vi "Auto_calibrate.vi"(3 "Mode":T4, 5 "Traverse line":T5 {"Carrier_2 Q (l/min)" format="%#.2f"; "Row Duration (mins)" format="%#.1f"; "Row No" min=0; "Trace Gas Concentration (%)" min=0.0 format="%#_4f"; "Carrier_1 Q (l/min)" format="%#.2f"; "Tunnel Speed" format="%#.2f"; "Start X" format="%#.2f"; "Start Y" format="%#.2f"; "Start Z" format="%#.2f"; "End X" format="%#.2f"; "End Y" format="%#.2f"; "End Z" format="%#.2f"; "Averaging time (min)" min=0.0 format="%#.2f"}) -> (0 "Error Messages":string, 1 "Status":T2, 2 "Traverse Out":T5 {"Carrier_2 Q (l/min)" format="%#.2f"; "Row Duration (mins)" format="%#.1f"; "Row No" min=0; "Trace Gas Concentration (%)" min=0.0 format="%#_4f"; "Carrier_1 Q (l/min)" format="%#.2f"; "Tunnel Speed" format="%#.2f"; "Start X" format="%#.2f"; "Start Y" format="%#.2f"; "Start Z" format="%#.2f"; "End X" format="%#.2f"; "End Y" format="%#.2f"; "End Z" format="%#.2f"; "Averaging time (min)" min=0.0 format="%#.2f"})   [LabVIEW 2014]
uses:
  Gen Trav/Traverse_cluster.ctl
  Gen Trav/Spacing.ctl
  Controls/Multi_run_mode.ctl
  Controls/User_Specific_mode.ctl
  Controls/Auto_Calib_Type.ctl
  Gen Trav/Multi_Run_Status.ctl
  Controls/Auto_Calib_Case.ctl
  File/Setup_Filetype.ctl
  Calibration/Calib_mode.ctl
  ADAM Client/Sub VIs/ADAM Controls/Valco_valve_ph.ctl
  ADAM Client/Sub VIs/ADAM Controls/Client_Source_Status.ctl
  Controls/Setup.ctl
  Controls/Post_Process.ctl
  Controls/Save_Data.ctl
  Controls/App_Global.ctl
  <vilib>/Analysis/baseanly.llb/Mean (DBL).vi
  Globals/Preference_global.vi
  Globals/Meas_global.vi
  Globals/Calib_global.vi
  Globals/Trav_pos_global.vi
  Globals/Gas_management_global.vi
  Globals/Extra_Commands_Global.vi
  <vilib>/Analysis/NI_AALBase.lvlib
  <vilib>/Analysis/NI_AALPro.lvlib
panel:
  out "Mix_own_Calib_Gases":bool
  out "Slope":dbl[](array[numeric])
  out "Minimum St Dev":dbl[](array[numeric])
  out "Wait factor":dbl
  out "Orig Calib file string":string
  out "Concentrations":dbl[](array[numeric])
  out "FFID St Dev":dbl[][](array[numeric]) format="%.2f"
  in  "Clear Calib History":bool
  out "Coefficients":dbl[][](array[numeric]) format="%.2f"
  out "Currently in Case":T1
  out "Valve position":dbl format="%.2f"
  out "Currently On":i32
  out "Values":dbl[][](array[numeric]) format="%.2f"
  out "FF Indexes":i16[](array[numeric])
  out "Ch No's":i16[](array[numeric])
  out "No of Calib Points":i32
  out "Root Name":string[](array[string])
  out "Calibration varying":T3
  in  "stop":bool
  out "New Calib Filenames":path[](array[path])
  # "Specific Argument Options\n      Tunnel Speed;1;2;3;4\nOR  Traverse Position\nOR   Concentration"
  # "X           Y            Z"
  # "Start"
  # "End"
  # "X           Y            Z"
  # "Start"
  # "End"
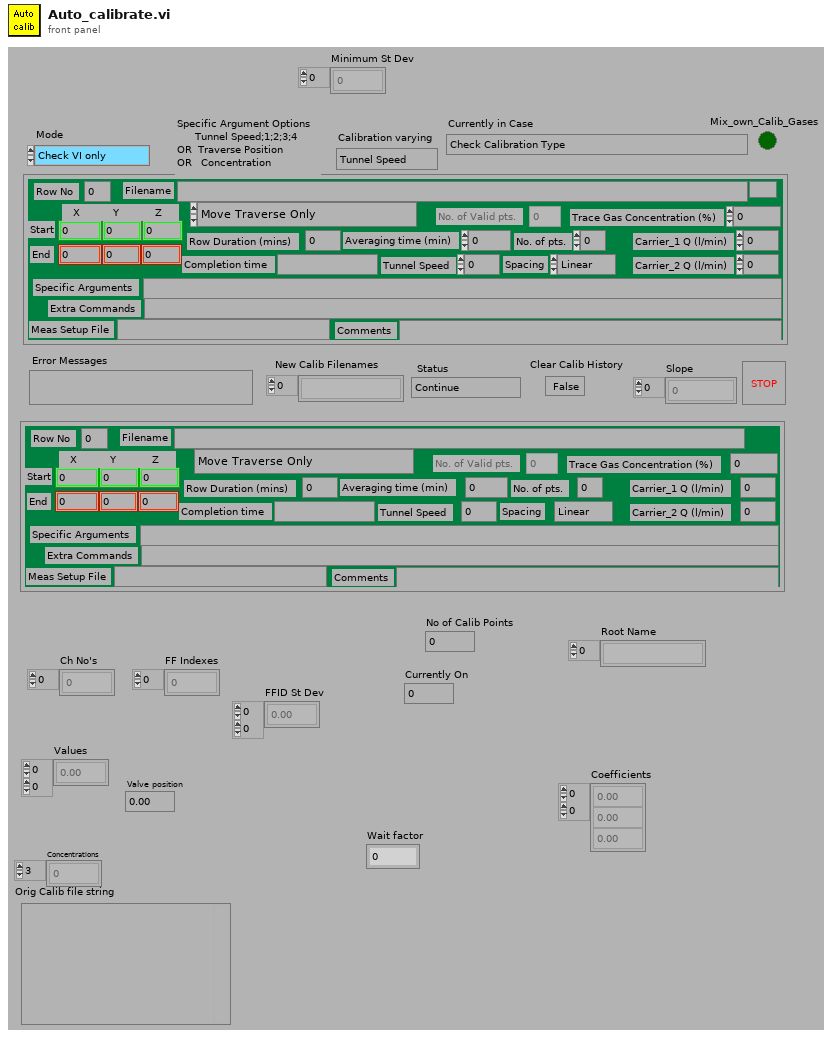
[diagram p1: front panel]
types:
  T1 = typedef "Auto_Calib_Case.ctl" = enum16{"Check Calibration Type", "Check if Original Calib file is Valid", "Get sampling rate etc. from meas setup file", "Setup Calibration Program", "Get Channel Numbers", "Check use latest selected on Mesurement setup files", "Create New Calib Filenames", "Setup Calibration Values in 2D array", "Create Measurement Setup File (Concentration Only)", "Are There Enough Calibration Points", "Set Measurement Conditions", "Measure Calibration Point", "Do Another Calibration Point?", "Skip Next Frame?", "Insert New calibration Filenames into Measurement Setup file", "Warn if FFID calibration is very non linear", "Warn if FFID variance is high", "Insert Bkgnd Variance into calib file", "Warn if FFID voltages are too low", "Warn if Current Calibration fit is poor", "Warn if Calibration Coefficients have significantly altered", "End"}
  T2 = typedef "Multi_Run_Status.ctl" = enum16{"Continue", "Jump to Next Point", "Jump to Next Row", "Jump To Fall Back", "Terminate Run"}
  T3 = typedef "Auto_Calib_Type.ctl" = enum16{"Tunnel Speed", "Traverse Position", "Concentration"}
  T4 = typedef "User_Specific_mode.ctl" = enum16{"Check VI only", "Run VI"}
  T5 = typedef "Traverse_cluster.ctl" = cluster{"Start X":sgl, "Start Y":sgl, "Start Z":sgl, "End X":sgl, "End Y":sgl, "End Z":sgl, "No. of pts.":i32, "Spacing":T6, "Filename":path, "Tunnel Speed":dbl, "Averaging time (min)":dbl, "Extra Commands":string, "Carrier_1 Q (l/min)":dbl, "Carrier_2 Q (l/min)":dbl, "Trace Gas Concentration (%)":dbl, "Specific Arguments":string, "Comments":string, "Row No":i32, "Row Type Selector":T7, "Completion time":string, "Row Duration (mins)":dbl, "No. of Valid pts.":i32, "Meas Setup File":string}
  T6 = typedef "Spacing.ctl" = enum16{"Linear", "Log", "Gauss", "Specified", "N/A"}
  T7 = typedef "Multi_run_mode.ctl" = enum16{"Move Traverse Only", "Set Tunnel Speed Only", "Set Source Only", "Set Measurement Conditions", "Single Measurement", "Vertical Profile", "Lateral Profile", "Longitudinal Profile", "Explore Volume", "Multi-Axis Profile", "Auto Calibrate", "Meas Fast FID Bkgnd", "Check Beam Power", "Scanning Valve Measurement", "Run VI Named:", "Set ADAM Ch", "Wait (minutes)", "Send Message", "Synchronize With:", "Fall Back to this Row", "Turn Off Row Repeating", "Blank Row", "Traverse 3D Volume"}
  T8 = typedef "Setup_Filetype.ctl" = enum16{"Measurement Setups", "Calibration Setups", "General", "Results File Plotter Setups", "Speed Calib Tweaks"}
  T9 = typedef "Calib_mode.ctl" = enum16{"Show Setup", "Take a New Calibration Point", "Refit Curve", "Setup Front Panel"}
  T10 = typedef "Client_Source_Status.ctl" = enum16{"Not Using", "Using", "Must Have"}
  T11 = typedef "Save_Data.ctl" = enum16{"Save No Data", "Save Data"}
  T12 = typedef "Post_Process.ctl" = enum16{"Take New Data", "Post Process Raw Data File"}
  T13 = typedef "Setup.ctl" = enum16{"Run Program", "Show Setup", "Save Current Setup", "Setup Front Panel"}
  T14 = typedef "App_Global.ctl" = enum16{"Read Global", "Write to Global", "Initialise Array"}
  T15 = typedef "Cal_Inst_type.ctl" = enum16{"Propeller anemometer", "Pressure Transducer", "Hot wire", "Cross wire velocity", "Cross wire angle", "Generic Linear", "Generic Polynomial", "Generic BackPoly", "Fast FID", "Thermocouple", "Cold wire", "Pulsed Wire"}
  T16 = typedef "Ref_Inst_type.ctl" = enum16{"Propellor anemometer", "Pressure Transducer", "Raw voltage", "Pitot-static tube", "Preston tube", "Generic Linear", "Generic Polynomial", "Thermocouple", "LDA", "Enter Value", "ADAM Channel"}
  T17 = cluster{"2nd Ref type":T16, "2nd inst present":bool}
  T18 = cluster{"high limit (10V)":sgl, "low limit (-10V)":sgl, "Ch No":i16, "Var name":string}[]
  T19 = cluster{"high limit (10V)":sgl, "low limit (-10V)":sgl, "Ch No":i16, "Var name":string}
  T20 = typedef "Inst_type.ctl" = enum16{"Propeller anemometer", "Raw voltage", "Pressure Transducer", "Pitot-static tube", "Preston tube", "Hot wire", "Cross wire 1", "Cross wire 2", "Generic Linear", "Generic Polynomial", "Generic BackPoly", "Fast FID", "Thermocouple", "Cold wire", "Pulsed Wire", "LDA Vel", "LDA Tran time", "LDA Arr time", "Microphone"}
  T21 = cluster{"high limit (10V)":sgl, "low limit (-10V)":sgl, "Ch No":i16, "Calib filename":path, "Inst type":T20, "Symbol":string, "Move channel":bool, "Use Latest":bool, "D":dbl, "Ch Name":string}[]
  T22 = typedef "Valco_valve_ph.ctl" = u16
  T23 = typedef "Status_Cluster.ctl" = cluster{"Status":T2, "Error Type":string, "Error Description":string}
  T24 = typedef "Time_Trace_Cluster.ctl" = cluster{"Weighting":dbl[], "Time (s)":dbl[], "Voltage":dbl[], "Eng Values":dbl[]}
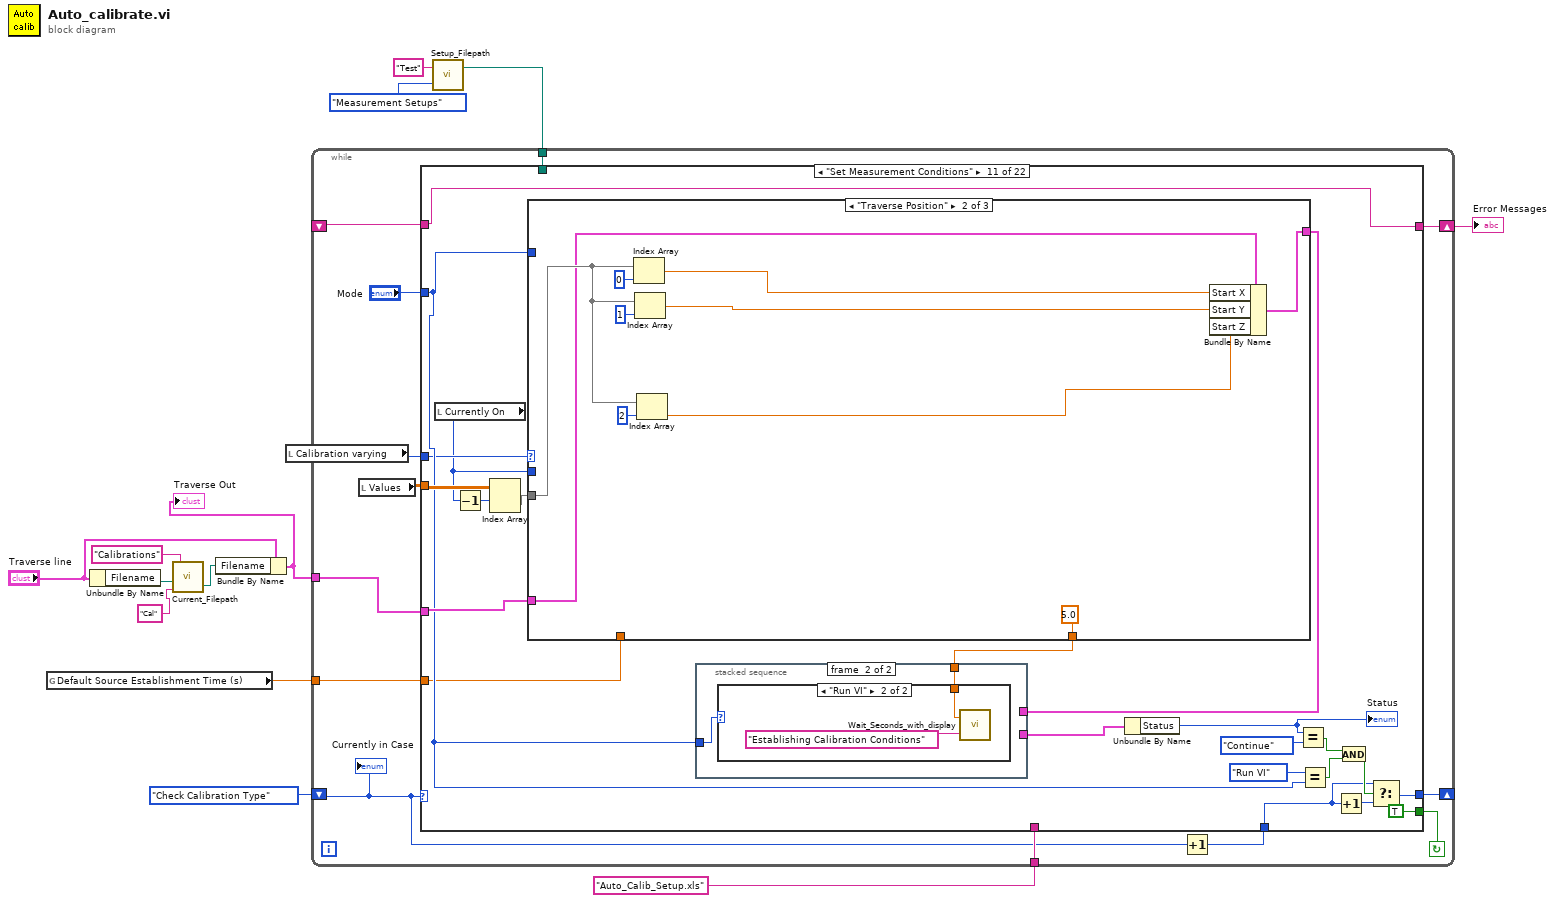
[diagram p0: block diagram]
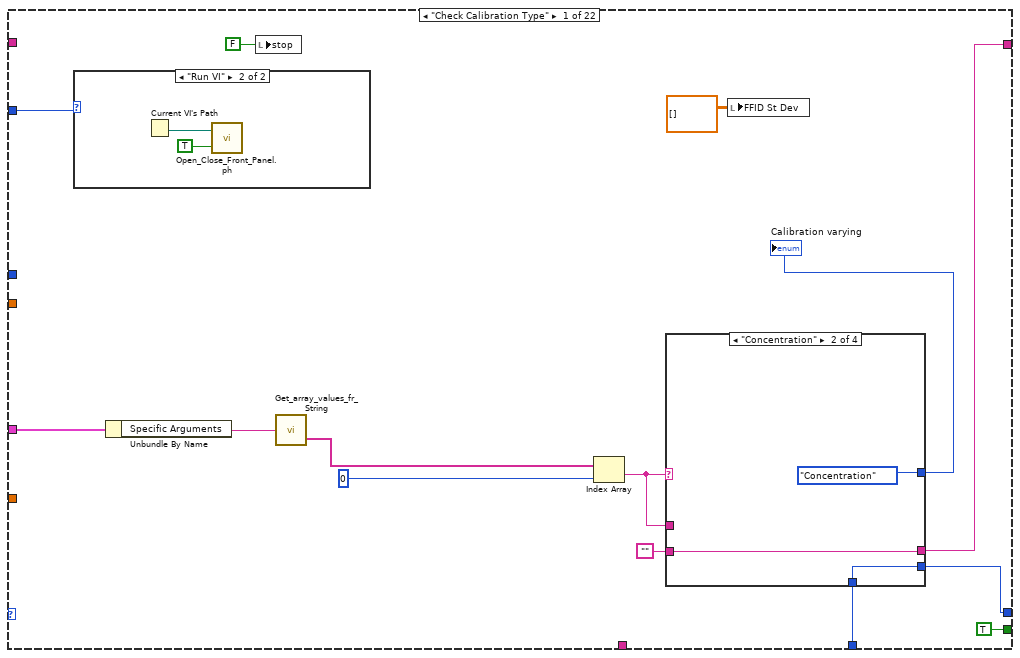
[diagram p2: hidden frame]
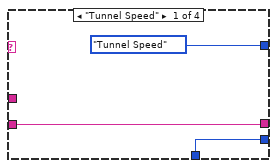
[diagram p4: hidden frame]
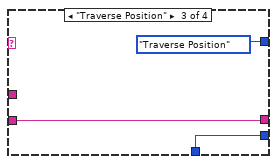
[diagram p5: hidden frame]
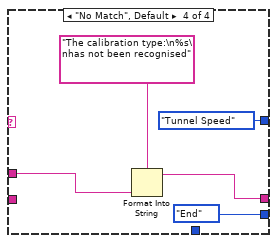
[diagram p6: hidden frame]
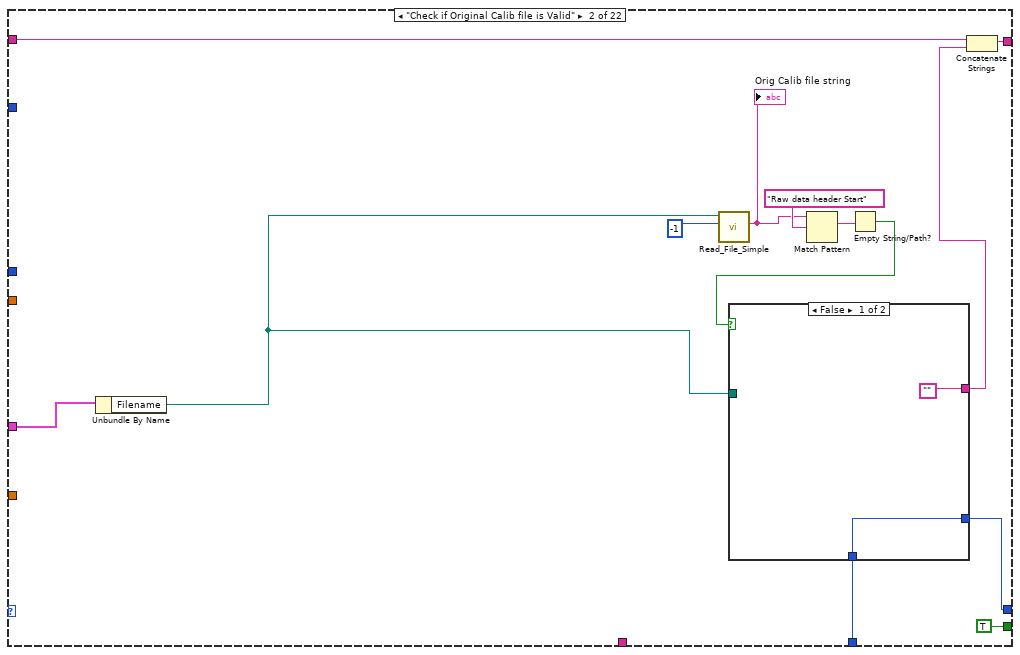
[diagram p7: hidden frame]
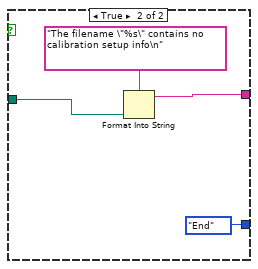
[diagram p8: hidden frame]
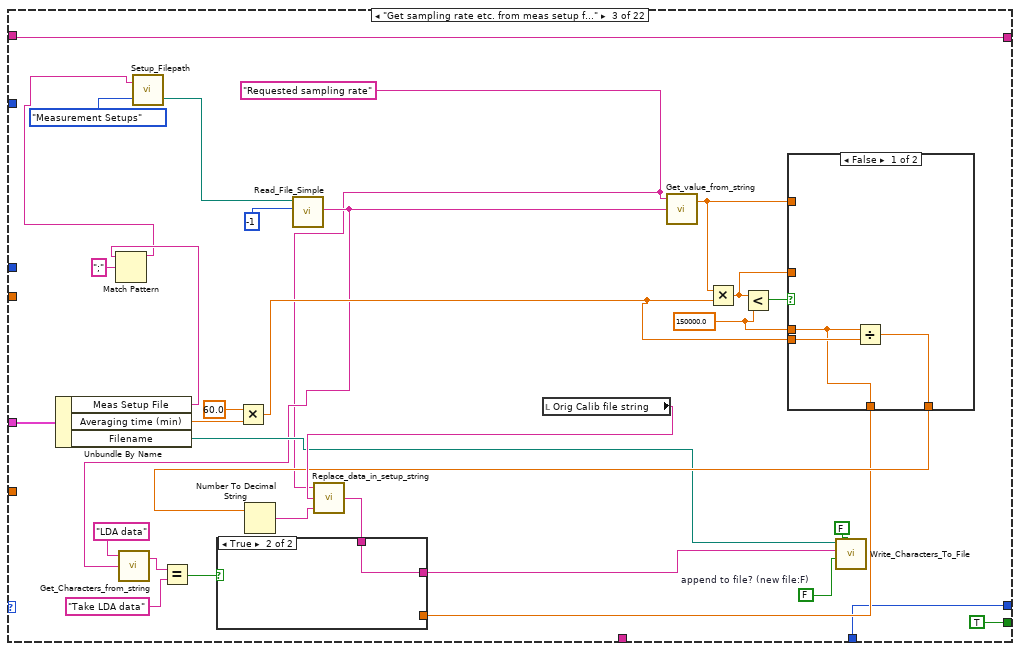
[diagram p9: hidden frame]
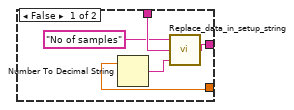
[diagram p10: hidden frame]
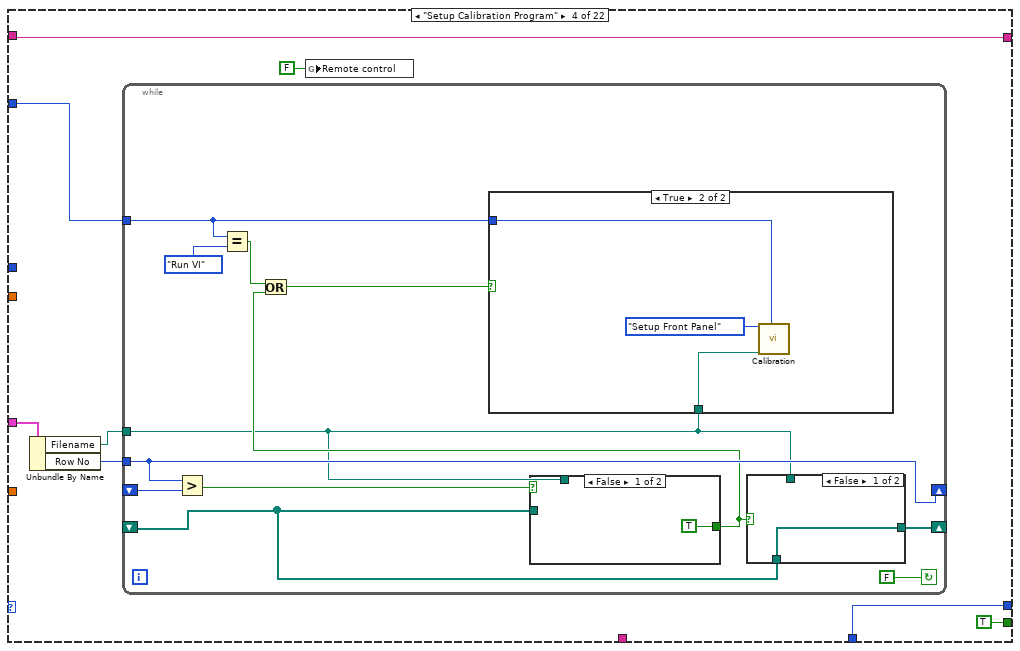
[diagram p12: hidden frame]
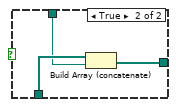
[diagram p13: hidden frame]
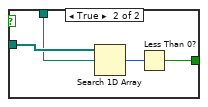
[diagram p15: hidden frame]
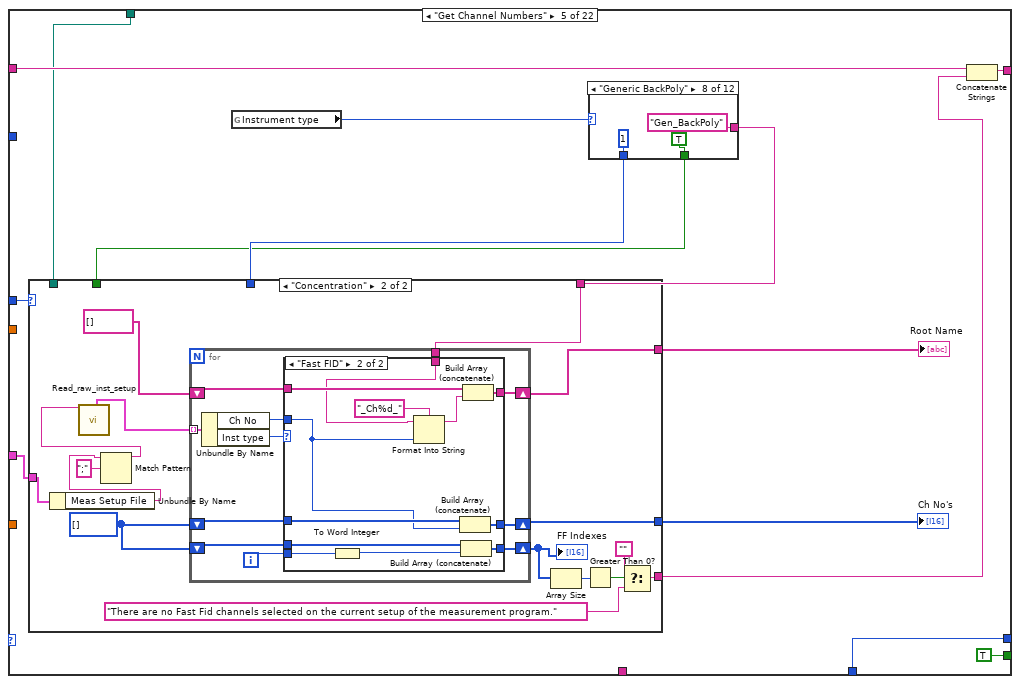
[diagram p16: hidden frame]
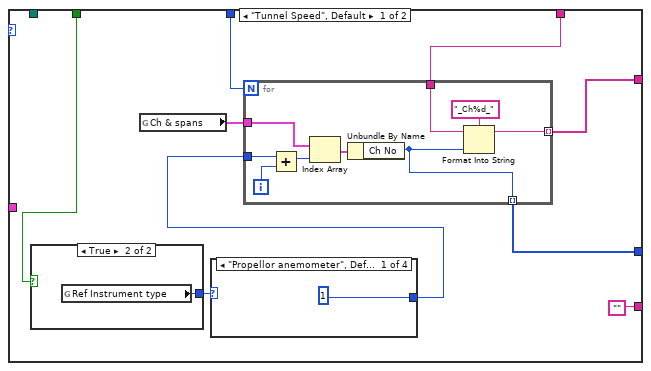
[diagram p17: hidden frame]
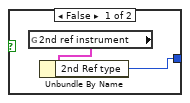
[diagram p18: hidden frame]
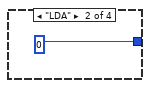
[diagram p19: hidden frame]
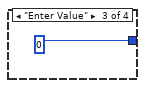
[diagram p20: hidden frame]
diagram:
  n1 = global read "Preference_global.vi" "Default Source Establishment Time (s)"() -> (w1:dbl)
  n2 = Unbundle By Name("Traverse line") -> ("Filename"=w6:path)
  n3 = call "Current_Filepath.vi"("Short_Name"="Cal" ("Data Type"), "Filename in"=w6, "Data Type"="Calibrations") -> ("Filename Out"=w5:path)  [unwired: 1 in, 1 out]
  n4 = Bundle By Name(cluster="Traverse line", "Filename"=w5) -> (w3:T5)
  "Traverse Out" <- w3
  n5 = call "Setup_Filepath.vi"("Setup File Type"=Setup_Filetype."Measurement Setups", "Filename in"="Test") -> ("Directory"=w8:path)  [unwired: 1 out]
  n6 = while {
    shift-left: _ -> [w19]
    shift-right: [w20] -> w12
    shift-left: Auto_Calib_Case."Check Calibration Type" ("Currently in Case") -> [w18]
    shift-right: [w17] -> _
    tunnel: "Auto_Calib_Setup.xls" -> [w26]
    tunnel: w8 -> [w16]
    tunnel: w3 -> [w15]
    tunnel: w1 -> [w14]
    stop <- w23 continue-if-true
    n7 = local read "Calibration varying"() -> (w22:T3)
    n8 = local read "Values"() -> (w21:dbl[][])
    n9 = Increment(x=w18) -> (x+1=w24:T1)
    n10 = case shown="\"Set Measurement Conditions\"" w18 {
      tunnel: w15 -> [w40 w69 w107 w122 w153 _ w321 w375 w432 _ w645 _ _ _ _ _ _ _ _ _ w1116 w1147]
      tunnel: "Mode" -> [w31 _ _ w123 _ _ w327 _ w433 _ w640 _ w862 w887 _ _ _ _ _ _ _ w1148]
      tunnel: w26 -> [_ _ _ _ _ _ _ _ w436 _ _ w732 _ _ _ _ _ _ _ _ _ _]
      tunnel: [w29 w59 w89 w125 w156 w272 w325 w367 w428 w608 w633 w731 w863 w890 w902 w921 w959 w1024 w1040 w1095 w1139 w1152] -> w17
      tunnel: w24 -> [w30 w58 w89 w125 w156 w272 w325 w368 w427 w607 w629 w731 _ w889 w901 w921 w959 w1024 w1040 w1095 w1139 w1152]
      tunnel: [TRUE TRUE TRUE TRUE TRUE TRUE TRUE TRUE TRUE TRUE TRUE TRUE TRUE TRUE TRUE TRUE TRUE TRUE TRUE TRUE TRUE FALSE] -> w23
      tunnel: w22 -> [_ _ _ _ w160 _ w324 w373 _ _ w632 w733 w861 w888 w904 _ _ _ _ _ _ w1149]
      tunnel: w21 -> [_ _ _ _ _ _ _ _ w431 w617 w644 _ _ _ _ _ w966 _ _ _ _ w1146]
      tunnel: [w33 w61 w87 w126 w157 w273 w337 w370 w435 w611 w630 w729 w860 w893 w908 w930 w973 w1020 w1045 w1084 w1132 w1151] -> w20
      tunnel: w19 -> [_ w63 w87 w126 w159 w273 w337 w369 w435 w612 w630 w729 w860 w893 w908 w930 w973 w1020 w1045 w1084 w1132 w1151]
      tunnel: w16 -> [_ _ _ _ w152 w275 _ _ w434 _ _ _ _ _ _ _ _ _ _ _ _ _]
      tunnel: w14 -> [_ _ _ _ _ _ _ _ w430 _ w627 _ _ _ _ _ _ _ _ _ _ _]
      frame "Check Calibration Type" {
        n11 = case shown="\"Run VI\"" w31 {
          frame "Check VI only" {
          }
          frame "Run VI" {
            n12 = Current VI's Path() -> (path=w41:path)
            n13 = call "Open_Close_Front_Panel.ph.vi"("Front Panel Window:Open"=TRUE, "VI path"=w41) -> ()  [unwired: 2 out]
          }
        }
        n14 = Unbundle By Name(w40) -> ("Specific Arguments"=w39:string)
        n15 = local write "stop"(FALSE) -> ()
        n16 = call "Get_array_values_fr_String.vi"("String Value"=w39) -> ("String array"=w38:string[])  [unwired: 1 out]
        n17 = Index Array(array=w38, index=0 ("Index")) -> (element=w36:string)
        n18 = case shown="\"Concentration\"" w36 {
          tunnel: [Auto_Calib_Type."Tunnel Speed" ("Calibration varying") Auto_Calib_Type."Concentration" ("Calibration varying") Auto_Calib_Type."Traverse Position" ("Calibration varying") Auto_Calib_Type."Tunnel Speed" ("Calibration varying")] -> w34
          tunnel: w36 -> [_ _ _ w55]
          tunnel: [w44 w47 w50 w53] -> w33
          tunnel: "" -> [w44 w47 w50 _]
          tunnel: w30 -> [w43 w46 w49 _]
          tunnel: [w43 w46 w49 Auto_Calib_Case."End" ("Currently in Case")] -> w29
          frame "Tunnel Speed" {
          }
          frame "Concentration" {
            (unwired) ""
          }
          frame "Traverse Position" {
          }
          frame "No Match", Default {
            n19 = Format Into String(format string="The calibration type:\n%s\nhas not been recognised" ("Format String"), w55) -> (resulting string=w53:string)  [unwired: 2 in, 1 out]
          }
        }
        "Calibration varying" <- w34
        n20 = local write "FFID St Dev"(dbl[][] [] ("FFID Variance")) -> ()
      }
      frame "Check if Original Calib file is Valid" {
        n21 = Unbundle By Name(w69) -> ("Filename"=w57:path)
        n22 = call "Read_File_Simple.vi"("Filename"=w57, "number of characters (all:-1)"=-1) -> ("string"=w66:string)  [unwired: 1 in, 7 out]
        "Orig Calib file string" <- w66
        n23 = Match Pattern(string=w66, regular expression="Raw data header Start") -> (match substring=w65:string)  [unwired: 4 out]
        n24 = Empty String/Path?(string/path=w65) -> (empty?=w64:bool)
        n25 = case shown="False" w64 {
          tunnel: w57 -> [_ w75]
          tunnel: ["" w73] -> w62
          tunnel: [w70 Auto_Calib_Case."End" ("Currently in Case")] -> w59
          tunnel: w58 -> [w70 _]
          frame False {
          }
          frame True {
            n26 = Format Into String(format string="The filename \"%s\" contains no calibration setup info\n" ("Format String"), w75) -> (resulting string=w73:string)  [unwired: 2 in, 1 out]
          }
        }
        n27 = Concatenate Strings(w63, w62) -> (w61:string)
      }
      frame "Get sampling rate etc. from meas setup file" {
        w90 = FALSE  # append to file? (new file:F)
        w79 = "Requested sampling rate"
        w97 = 150000.0 ("y")
        n28 = Unbundle By Name(w107) -> ("Meas Setup File"=w85:string, "Averaging time (min)"=w105:dbl, "Filename"=w92:path)
        n29 = Match Pattern(string=w85, regular expression=";") -> (before substring=w77:string)  [unwired: 4 out]
        n30 = call "Setup_Filepath.vi"("Setup File Type"=Setup_Filetype."Measurement Setups", "Filename in"=w77) -> ("Filename Out"=w76:path)  [unwired: 1 out]
        n31 = Multiply(x=60.0, y=w105) -> (x*y=w96:dbl)
        n32 = call "Read_File_Simple.vi"("Filename"=w76, "number of characters (all:-1)"=-1) -> ("string"=w84:string)  [unwired: 1 in, 7 out]
        n33 = call "Get_Characters_from_string.vi"("Input string"=w84, "Variable name"="LDA data") -> ("Value"=w82:string)  [unwired: 1 in, 1 out]
        n34 = Equal?(x=w82, y="Take LDA data") -> (x = y?=w80:bool)
        n35 = local read "Orig Calib file string"() -> (w101:string)
        n36 = call "Get_value_from_string.vi"("Input string"=w84, "Variable name"=w79) -> ("Value"=w100:dbl)  [unwired: 1 in, 1 out]
        n37 = Multiply(x=w100, y=w96) -> (x*y=w95:dbl)
        n38 = Less?(x=w95, y=w97) -> (x < y?=w103:bool)
        n39 = case shown="False" w103 {
          tunnel: w100 -> [_ w118]
          tunnel: [w115 w118] -> w99
          tunnel: w97 -> [w114 _]
          tunnel: w96 -> [w116 _]
          tunnel: [w114 w117] -> w93
          tunnel: w95 -> [_ w117]
          frame False {
            n40 = Divide(x=w114, y=w116) -> (x/y=w115:dbl)
          }
          frame True {
          }
        }
        n41 = Number To Decimal String(number=w99) -> (decimal integer string=w98:string)  [unwired: 1 out]
        n42 = call "Replace_data_in_setup_string.vi"("New data string"=w98, "Input string"=w101, "Variable name"=w79) -> ("Appended string"=w94:string)
        n43 = case shown="True" w80 {
          tunnel: w94 -> [w112 w113]
          tunnel: w93 -> [w109 _]
          tunnel: [w108 w113] -> w91
          frame False {
            n44 = Number To Decimal String(number=w109) -> (decimal integer string=w110:string)  [unwired: 1 out]
            n45 = call "Replace_data_in_setup_string.vi"("New data string"=w110, "Input string"=w112, "Variable name"="No of samples") -> ("Appended string"=w108:string)
          }
          frame True {
          }
        }
        n46 = call "Write_Characters_To_File.vi"("file path (dialog if empty)"=w92, "advisory dialog? (display:T)"=FALSE, "character string"=w91, "append to file? (new file:F)"=w90) -> ()  [unwired: 1 in, 4 out]
      }
      frame "Setup Calibration Program" {
        n47 = Unbundle By Name(w122) -> ("Filename"=w119:path, "Row No"=w121:i32)
        n48 = while {
          shift-left: _ -> [w130]
          shift-right: [w129] -> _
          tunnel: w121 -> [w137]
          shift-left: _ -> [w138]
          shift-right: [w137] -> _
          tunnel: w123 -> [w135]
          tunnel: w119 -> [w127]
          stop <- FALSE continue-if-true
          n49 = Greater?(x=w137, y=w138) -> (0:w136:bool)
          n50 = Equal?(x=w135, y=User_Specific_mode."Run VI" ("Mode")) -> (x = y?=w133:bool)
          n51 = case shown="False" w136 {
            tunnel: w130 -> [_ w150]
            tunnel: w127 -> [_ w149]
            tunnel: [TRUE w147] -> w131
            frame False {
            }
            frame True {
              n52 = Search 1D Array(1D array=w150, element=w149) -> (index of element=w148:i32)  [unwired: 1 out]
              n53 = Less Than 0?(x=w148) -> (x < 0?=w147:bool)
            }
          }
          n54 = Or(x=w133, y=w131) -> (x .or. y?=w132:bool)
          n55 = case shown="True" w132 {
            tunnel: w135 -> [_ w145]
            tunnel: w127 -> [_ w144]
            frame False {
            }
            frame True {
              n56 = call "Calibration.vi"("Mode"=Calib_mode."Setup Front Panel", "Calib file"=w144, "Simulate/Run"=w145) -> ()  [unwired: 17 out]
            }
          }
          n57 = case shown="False" w131 {
            tunnel: w130 -> [w139 w142]
            tunnel: w127 -> [_ w141]
            tunnel: [w139 w140] -> w129
            frame False {
            }
            frame True {
              n58 = Build Array (concatenate)(w142, w141) -> (w140:path[])
            }
          }
        }
        n59 = global write "Meas_global.vi" "Remote control"(FALSE ("Remote control")) -> ()
      }
      frame "Get Channel Numbers" {
        n60 = global read "Calib_global.vi" "Instrument type"() -> (w164:T15)
        n61 = case shown="\"Generic BackPoly\"" w164 {
          tunnel: ["Prop" "Mano" "HW" "XW" "XW" "Gen_Lin" "Gen_Poly" "Gen_BackPoly" "FF" "Therm" "CW" "PWA"] -> w163
          tunnel: [1 1 1 2 2 1 1 1 1 1 1 1] -> w154
          tunnel: [TRUE TRUE TRUE TRUE FALSE TRUE TRUE TRUE TRUE TRUE TRUE TRUE] -> w151
          frame "Propeller anemometer" {
          }
          frame "Pressure Transducer" {
          }
          frame "Hot wire" {
          }
          frame "Cross wire velocity" {
          }
          frame "Cross wire angle" {
          }
          frame "Generic Linear" {
          }
          frame "Generic Polynomial" {
          }
          frame "Generic BackPoly" {
          }
          frame "Fast FID" {
          }
          frame "Thermocouple" {
          }
          frame "Cold wire" {
          }
          frame "Pulsed Wire" {
          }
        }
        n62 = case shown="\"Concentration\"" w160 {
          tunnel: w163 -> [w171 w205]
          tunnel: [w167 w204] -> w162
          tunnel: [w168 w202] -> w161
          tunnel: ["" w195] -> w158
          tunnel: w154 -> [w169 _]
          tunnel: w153 -> [_ w194]
          tunnel: w152 -> [_ _]
          tunnel: w151 -> [w165 _]
          frame "Tunnel Speed", Default {
            n63 = case shown="True" w165 {
              tunnel: [w174 w176] -> w173
              frame False {
                n64 = global read "Calib_global.vi" "2nd ref instrument"() -> (w175:T17)
                n65 = Unbundle By Name(w175) -> ("2nd Ref type"=w174:T16)
              }
              frame True {
                n66 = global read "Calib_global.vi" "Ref Instrument type"() -> (w176:T16)
              }
            }
            n67 = global read "Calib_global.vi" "Ch & spans"() -> (w170:T18)
            n68 = case shown="\"Propellor anemometer\", Default" w173 {
              tunnel: [1 i16 0 0 0] -> w166
              frame "Propellor anemometer", Default {
              }
              frame "LDA" {
              }
              frame "Enter Value" {
              }
              frame "ADAM Channel" {
              }
            }
            n69 = for {
              N: w169 -> [_]
              tunnel: [w183] -> w168 mode=indexing
              tunnel: w171 -> [w182]
              tunnel: w170 -> [w181]
              tunnel: [w180] -> w167 mode=indexing
              tunnel: w166 -> [w178]
              i -> [w179]
              n70 = Add(x=w178, y=w179) -> (x+y=w177:i32)
              n71 = Index Array(array=w181, index=w177) -> (element=w185:T19)
              n72 = Unbundle By Name(w185) -> ("Ch No"=w183:i16)
              n73 = Format Into String(format string="_Ch%d_" ("Format String"), initial string=w182, w183) -> (resulting string=w180:string)  [unwired: 1 in, 1 out]
            }
          }
          frame "Concentration" {
            w201 = i16[] []
            n74 = Unbundle By Name(w194) -> ("Meas Setup File"=w191:string)
            n75 = Match Pattern(string=w191, regular expression=";") -> (before substring=w190:string)  [unwired: 4 out]
            n76 = call "Read_raw_inst_setup.vi"("Setup file"=w190) -> ("Ch & spans choices"=w193:T21)  [unwired: 18 out]
            n77 = for {
              tunnel: w193 -> [w216] mode=indexing
              tunnel: w205 -> [w215]
              shift-right: [w211] -> w204
              shift-left: string[] [] -> [w212]
              shift-right: [w209] -> w202
              shift-left: w201 -> [w210]
              shift-right: [w208] -> w200
              shift-left: w201 -> [w207]
              i -> [w206]
              n78 = Unbundle By Name(w216) -> ("Ch No"=w214:i16, "Inst type"=w213:T20)
              n79 = case shown="\"Fast FID\"" w213 {
                tunnel: w215 -> [_ w221]
                tunnel: w214 -> [_ w223]
                tunnel: w212 -> [w219 w231]
                tunnel: [w219 w230] -> w211
                tunnel: w210 -> [w218 w229]
                tunnel: [w218 w228] -> w209
                tunnel: w207 -> [w217 w226]
                tunnel: [w217 w227] -> w208
                tunnel: w206 -> [_ w225]
                frame "Generic Linear", Default {
                }
                frame "Fast FID" {
                  n80 = To Word Integer(number=w225) -> (16bit integer=w224:i16)
                  n81 = Format Into String(format string="_Ch%d_", initial string=w221, w223) -> (resulting string=w220:string)  [unwired: 1 in, 1 out]
                  n82 = Build Array (concatenate)(w229, w223) -> (w228:i16[])
                  n83 = Build Array (concatenate)(w226, w224) -> (w227:i16[])
                  n84 = Build Array (concatenate)(w231, w220) -> (w230:string[])
                }
              }
            }
            "FF Indexes" <- w200
            n85 = Array Size(array=w200) -> (size(s)=w199:i32)
            n86 = Greater Than 0?(x=w199) -> (x > 0?=w198:bool)
            n87 = Select(t="", s=w198, f="There are no Fast Fid channels selected on the current setup of the measurement program.") -> (s? t:f=w195:string)
          }
        }
        "Root Name" <- w162
        "Ch No's" <- w161
        n88 = Concatenate Strings(w159, w158) -> (w157:string)
      }
      frame "Check use latest selected on Mesurement setup files" {
        n89 = global read "Trav_pos_global.vi" "Measurement setup files"() -> (w268:string[])
        n90 = local read "Ch No's"() -> (w274:i16[])
        n91 = Build Array (concatenate)(w268, "Current_Setup.xls") -> (w269:string[])
        n92 = for {
          tunnel: w275 -> [w278]
          tunnel: w269 -> [w277] mode=indexing
          tunnel: w274 -> [w276]
          n93 = stacked-sequence {
            seq-local: [w279 _ _] -> [_ w285 w313]
            seq-local: [_ w283 _] -> [_ _ w311]
            tunnel: w278 -> [w282 _ w310]
            tunnel: w277 -> [w281 _ w309]
            tunnel: w276 -> [_ w284 _]
            frame #0 {
              n94 = Build Path(base path=w282, name or relative path=w281) -> (appended path=w280:path)
              n95 = call "Read_File_Simple.vi"("Filename"=w280) -> ("string"=w279:string)  [unwired: 2 in, 7 out]
            }
            frame #1 {
              n96 = while {
                shift-right: [w290] -> w283
                shift-left: w285 -> [w291]
                tunnel: w284 -> [w294]
                i -> [w298]
                stop <- w287 continue-if-true
                n97 = Increment(x=w298) -> (x+1=w292:i32)
                n98 = Format Into String(format string="An ch %d Ch No", w292) -> (resulting string=w297:string)  [unwired: 2 in, 1 out]
                n99 = call "Get_value_from_string.vi"("Input string"=w291, "Variable name"=w297) -> ("Status"=w296:enum16{"Char in string", "Char not in string"}, "Value"=w295:dbl)  [unwired: 1 in]
                n100 = To Long Integer(number=w295) -> (32bit integer=w293:i32)
                n101 = Search 1D Array(1D array=w294, element=w293) -> (index of element=w289:i32)  [unwired: 1 in]
                n102 = Greater Or Equal To 0?(x=w289) -> (x >= 0?=w288:bool)
                n103 = case shown="\"Char in string\"" w296 {
                  tunnel: [TRUE FALSE] -> w287
                  frame "Char in string" {
                  }
                  frame "Char not in string" {
                  }
                }
                n104 = And(x=w288, y=w287) -> (x .and. y?=w286:bool)
                n105 = case shown="True" w286 {
                  tunnel: w292 -> [w302 _]
                  tunnel: w291 -> [w301 w306]
                  tunnel: [w300 w306] -> w290
                  frame True {
                    n106 = Format Into String(format string="An ch %d Use latest Calib", w302) -> (resulting string=w304:string)  [unwired: 2 in, 1 out]
                    n107 = call "Replace_data_in_setup_string.vi"("New data string"="TRUE" ("Replace with"), "Input string"=w301, "Variable name"=w304) -> ("Appended string"=w300:string)
                  }
                  frame False {
                  }
                }
              }
            }
            frame #2 {
              n108 = Equal?(x=w313, y=w311) -> (x = y?=w312:bool)
              n109 = case shown="True" w312 {
                tunnel: w310 -> [w316 _]
                tunnel: w311 -> [w319 _]
                tunnel: w309 -> [w315 _]
                frame False {
                  w318 = FALSE  # append to file? (new file:F)
                  n110 = Build Path(base path=w316, name or relative path=w315) -> (appended path=w314:path)
                  n111 = call "Write_Characters_To_File.vi"("file path (dialog if empty)"=w314, "advisory dialog? (display:T)"=FALSE, "character string"=w319, "append to file? (new file:F)"=w318) -> ()  [unwired: 1 in, 4 out]
                }
                frame True {
                }
              }
            }
          }
        }
      }
      frame "Create New Calib Filenames" {
        n112 = Unbundle By Name(w321) -> ("Filename"=w320:path)
        n113 = Get Date/Time String(date format (0)=enum16{"short", "long", "abbreviated"}."short") -> (date string=w331:string)  [unwired: 3 out]
        n114 = Strip Path(path=w320) -> (stripped path=w326:path)  [unwired: 1 out]
        n115 = local read "Root Name"() -> (w323:string[])
        n116 = case shown="\"Tunnel Speed\", Default" w324 {
          tunnel: w323 -> [_ w342]
          tunnel: [1 w341] -> w322
          frame "Tunnel Speed", Default {
          }
          frame "Concentration" {
            n117 = Array Size(array=w342) -> (size(s)=w341:i32)
          }
        }
        n118 = call "Replace_Character.vi"("Replace with"="-", "Input String"=w331, "Search For"="/") -> ("Output string"=w328:string)  [unwired: 1 out]
        n119 = List Folder(path=w326) -> (filenames=w339:string[])  [unwired: 1 in, 5 out]
        n120 = To Upper Case(1:w339) -> (0:w338:string[])
        n121 = for {
          N: w322 -> [_]
          tunnel: w323 -> [w345] mode=indexing
          tunnel: w338 -> [w349]
          tunnel: w326 -> [w348]
          tunnel: [w344] -> w335 mode=indexing
          tunnel: w328 -> [w346]
          tunnel: w327 -> [w343]
          n122 = while {
            tunnel: w345 -> [w356]
            tunnel: w346 -> [w357]
            tunnel: [w352] -> w347
            tunnel: w349 -> [w359]
            i -> [w361]
            stop <- w363 continue-if-true
            n123 = Increment(x=w361) -> (x+1=w358:i32)
            n124 = Format Into String(format string="%s_%d.xls" ("Format String"), initial string=w356, w357, w358) -> (resulting string=w353:string)  [unwired: 1 in, 1 out]
            n125 = call "Replace_Character.vi"("Replace with"="_", "Input String"=w353, "Search For"=" ") -> ("Output string"=w352:string)  [unwired: 1 out]
            n126 = To Upper Case(1:w352) -> (0:w362:string)
            n127 = Search 1D Array(1D array=w359, element=w362) -> (index of element=w364:i32)  [unwired: 1 out]
            n128 = Not Equal?(x=w364, y=-1) -> (x != y?=w363:bool)
          }
          n129 = Build Path(base path=w348, name or relative path=w347) -> (appended path=w344:path)
          n130 = case shown="\"Run VI\"" w343 {
            tunnel: w344 -> [_ w350]
            frame "Check VI only" {
            }
            frame "Run VI" {
              n131 = call "Calibration.vi"("Mode"=Calib_mode."Setup Front Panel", "Calib file"=w350) -> ()  [unwired: 1 in, 17 out]
            }
          }
        }
        "New Calib Filenames" <- w335
        n132 = Index Array(array=w335, index=0 ("Index")) -> (element=w333:path)
        n133 = global write "Meas_global.vi" "Results file"(w333) -> ()
      }
      frame "Setup Calibration Values in 2D array" {
        n134 = case shown="\"Concentration\"" w373 {
          tunnel: [w385 w395 w426] -> w372
          tunnel: w375 -> [w380 w393 w425]
          tunnel: ["" "" w424] -> w371
          tunnel: w368 -> [w379 w396 w423]
          tunnel: [w378 w396 w422] -> w367
          tunnel: [dbl[] [] w394 dbl[] []] -> w366
          frame "Tunnel Speed" {
            n135 = Unbundle By Name(w380) -> ("Specific Arguments"=w383:string)
            n136 = call "Get_array_values_fr_String.vi"("String Value"=w383) -> ("Numeric Array"=w381:dbl[])  [unwired: 1 out]
            n137 = Array Subset(array=w381, index=1 ("Array Index")) -> (w377:dbl[])  [unwired: 1 in]
            n138 = for {
              tunnel: w377 -> [w387] mode=indexing
              tunnel: [w386] -> w385 mode=indexing
              n139 = Build Array(w387) -> (w386:dbl[])
            }
            n140 = Increment(x=w379) -> (x+1=w378:T1)
          }
          frame "Concentration" {
            n141 = Unbundle By Name(w393) -> ("Specific Arguments"=w392:string)
            n142 = call "Read_FFID_Auto_Calib_Setup.vi"("Specific Argument"=w392) -> ("Trace concentration %"=w388:dbl[], "Carrier 2 Q"=w389:dbl[], "Carrier 1 Q"=w390:dbl[], "Mix_own_Calib_Gases"=w391:bool)  [unwired: 1 out]
            "Mix_own_Calib_Gases" <- w391
            n143 = case shown="True" w391 {
              tunnel: [w407 w416] -> w395
              tunnel: [w398 w411] -> w394
              tunnel: w390 -> [_ w415]
              tunnel: w389 -> [_ w414]
              tunnel: w388 -> [_ w413]
              frame False {
                w403 = 0.0 ("Input Element")
                n144 = Build Array(1.0, 2.0, 3.0) -> (w408:dbl[])
                n145 = Build Array("GMU:Calibration:Gas 1", "GMU:Calibration:Gas 2") -> (w399:string[])
                n146 = call "Get_Current_Scan_client.vi"("ADAM Ch Names"=w399) -> ("Numerical Values"=w402:dbl[])  [unwired: 3 out]
                n147 = Build Array (concatenate)(w403, w403, w402, w403) -> (w398:dbl[])
                n148 = for {
                  tunnel: w408 -> [w410] mode=indexing
                  tunnel: [w409] -> w407 mode=indexing
                  n149 = Build Array(w410) -> (w409:dbl[])
                }
              }
              frame True {
                n150 = for {
                  tunnel: w415 -> [w420] mode=indexing
                  tunnel: [w419] -> w416 mode=indexing
                  tunnel: w414 -> [w418] mode=indexing
                  tunnel: w413 -> [w417] mode=indexing
                  n151 = Build Array(w420, w418, w417) -> (w419:dbl[])
                }
                n152 = Multiply(x=10000.0, y=w413) -> (x*y=w411:dbl[])
              }
            }
          }
          frame "Traverse Position" {
            n153 = call "Create_Pos_array.vi"("Traverse line"=w425) -> ("Error Messages"=w424:string, "Array of Positions"=w426:dbl[][])  [unwired: 5 in, 2 out]
            n154 = Increment(x=w423) -> (x+1=w422:T1)
          }
        }
        "Values" <- w372
        "Concentrations" <- w366
        n155 = Concatenate Strings(w369, w371) -> (w370:string)
      }
      frame "Create Measurement Setup File (Concentration Only)" {
        n156 = stacked-sequence {
          seq-local: [_ w451 _ _ _ _ _ _] -> [_ _ w470 _ _ _ _ _]
          seq-local: [_ _ w468 _ _ _ _ _] -> [_ _ _ w491 _ _ _ _]
          seq-local: [_ _ _ _ w503 _ _ _] -> [_ _ _ _ _ _ _ w594]
          seq-local: [_ _ _ _ w499 _ _ _] -> [_ _ _ _ _ w540 _ _]
          tunnel: w434 -> [_ w442 _ w492 _ _ _ _]
          tunnel: w436 -> [_ _ _ w493 _ _ _ _]
          tunnel: w433 -> [_ _ _ _ w502 w539 w576 _]
          tunnel: w432 -> [_ w448 _ _ w500 _ _ _]
          tunnel: w431 -> [_ _ _ _ w504 _ _ _]
          tunnel: w430 -> [_ _ _ _ _ _ _ _]
          tunnel: [_ _ _ _ _ w538 _ _] -> w428
          tunnel: w427 -> [_ _ _ _ _ w537 _ _]
          frame #0 {
            n157 = global read "Gas_management_global.vi" "Source Live"() -> (w437:bool)
            n158 = case shown="True" w437 {
              frame False {
              }
              frame True {
                w438 = u32 1  # Time to hold source OFF (microseconds)
                w439 = u32 0  # Time to hold source ON (microseconds)
                n159 = call "Arduino_Timed_Release.vi"("Time to hold source ON (microseconds)"=w439, "Time to hold source OFF (microseconds)"=w438, "Number of cycles"=u16 1) -> ()  [unwired: 2 out]
              }
            }
          }
          frame #1 {
            w455 = TRUE  # Show Dialog?
            n160 = Unbundle By Name(w448) -> ("Meas Setup File"=w449:string)
            n161 = Match Pattern(string=w449, regular expression=";") -> (before substring=w447:string)  [unwired: 4 out]
            n162 = Build Path(base path=w442, name or relative path=w447) -> (appended path=w456:path)
            n163 = Format Into String(format string="Meas Setup File   %s", w442) -> (resulting string=w441:string)  [unwired: 2 in, 1 out]
            n164 = call "Read_spec_No_of_Characters.vi"("Filename"=w456) -> ("character string"=w457:string)  [unwired: 1 out]
            n165 = call "Get_string_subset.vi"("String Name"=w441, "Show Dialog?"=w455, "String to split"=w457, "File Label"="Raw data header") -> ("Output string"=w444:string)  [unwired: 1 out]
            n166 = call "Get_value_from_string.vi"("Input string"=w444, "Variable name"="No of analogue inst") -> ("Value"=w445:dbl)  [unwired: 1 in, 1 out]
            n167 = for {
              N: w445 -> [_]
              shift-right: [w459] -> w454
              shift-left: w444 -> [w461]
              i -> [w465]
              n168 = Increment(x=w465) -> (x+1=w464:i32)
              n169 = Number To Decimal String(number=w464) -> (decimal integer string=w467:string)  [unwired: 1 out]
              n170 = Concatenate Strings("An ch ", w467, " Inst type") -> (w462:string)
              n171 = call "Replace_data_in_setup_string.vi"("New data string"="Raw voltage", "Input string"=w461, "Variable name"=w462) -> ("Appended string"=w459:string)
            }
            n172 = call "Replace_data_in_setup_string.vi"("New data string"="No LDA data", "Input string"=w454, "Variable name"="LDA data" ("Label for characters")) -> ("Appended string"=w451:string)
          }
          frame #2 {
            n173 = global read "Calib_global.vi" "New Setup String"() -> (w471:string)
            n174 = for {
              N: 4 -> [_]
              shift-right: [w476] -> w468
              shift-left: w470 -> [w477]
              tunnel: w471 -> [w473]
              i -> [w475]
              n175 = case shown="3" w475 {
                tunnel: [w480 w483 w486 "No of blocks"] -> w474
                tunnel: w473 -> [w479 w482 w485 _]
                tunnel: [w478 w481 w484 "1" ("Value")] -> w472
                frame 0, Default {
                  w480 = "No of samples"
                  n176 = call "Get_Characters_from_string.vi"("Input string"=w479, "Variable name"=w480) -> ("Value"=w478:string)  [unwired: 1 in, 1 out]
                }
                frame 2 {
                  w483 = "Actual sampling rate"
                  n177 = call "Get_Characters_from_string.vi"("Input string"=w482, "Variable name"=w483) -> ("Value"=w481:string)  [unwired: 1 in, 1 out]
                }
                frame 3 {
                  w486 = "Board type"
                  n178 = call "Get_Characters_from_string.vi"("Input string"=w485, "Variable name"=w486) -> ("Value"=w484:string)  [unwired: 1 in, 1 out]
                }
                frame 1 {
                }
              }
              n179 = call "Replace_data_in_setup_string.vi"("New data string"=w472, "Input string"=w477, "Variable name"=w474) -> ("Appended string"=w476:string)
            }
          }
          frame #3 {
            w497 = FALSE  # advisory dialog? (display:T)
            w498 = FALSE  # append to file? (new file:F)
            n180 = call "Remove_Plug_Ins_etc.vi"("Input String"=w491) -> ("Output string"=w490:string)
            n181 = call "Add_label_to_string.vi"("String to write"=w490, "File Label"="Raw data header") -> ("Output string"=w494:string)
            n182 = Build Path(base path=w492, name or relative path=w493) -> (appended path=w489:path)
            n183 = call "Add_length_to_string.vi"("String in"=w494) -> ("String out"=w496:string)
            n184 = call "Write_Characters_To_File.vi"("file path (dialog if empty)"=w489, "advisory dialog? (display:T)"=w497, "character string"=w496, "append to file? (new file:F)"=w498) -> ()  [unwired: 1 in, 4 out]
          }
          frame #4 {
            n185 = local read "Mix_own_Calib_Gases"() -> (w501:bool)
            n186 = case shown="\"Run VI\"" w502 {
              tunnel: w504 -> [w509 _]
              tunnel: [w508 u32 0 ("millisecond timer value")] -> w503
              tunnel: w501 -> [w507 _]
              tunnel: w500 -> [w506 w536]
              tunnel: [w505 w536] -> w499
              frame "Run VI" {
                n187 = case shown="True" w507 {
                  tunnel: w509 -> [w512 w531]
                  tunnel: [w511 w526] -> w508
                  tunnel: w506 -> [w510 w528]
                  tunnel: [w510 w527] -> w505
                  frame False {
                    n188 = flat-sequence {
                      tunnel: w512 -> [w514]
                      tunnel: [w516] -> w511
                      frame #0 {
                        w515 = 0 ("Index")
                        n189 = Index Array(array=w514, index (row)=w515, index (col)=w515) -> (element=w513:dbl)
                        n190 = call "Fast_FID_Valve_Control.vi"("Requested Position"=w513) -> ()  [unwired: 7 out]
                      }
                      frame #1 {
                        n191 = Tick Count (ms)() -> (millisecond timer value=w516:u32)
                      }
                    }
                  }
                  frame True {
                    w532 = T22 4 items=["", "Zero Air", "Calib 1", "Calib 2", "Measure"] ("Requested Position")
                    n192 = Index Array(array=w531, index (row)=0) -> (element=w529:dbl[])  [unwired: 1 in]
                    n193 = flat-sequence {
                      tunnel: [w534] -> w526
                      frame #0 {
                        n194 = Wait (ms)(milliseconds to wait=u32 5000) -> ()  [unwired: 1 out]
                      }
                      frame #1 {
                        n195 = Tick Count (ms)() -> (millisecond timer value=w534:u32)
                      }
                    }
                    n196 = call "Fast_FID_Valve_Control.vi"("Requested Position"=w532) -> ()  [unwired: 7 out]
                    n197 = Index Array(array=w529) -> (element #1=w518:dbl, element #2=w519:dbl, element #3=w517:dbl)  [unwired: 3 in]
                    n198 = Bundle By Name(cluster=w528, "Carrier_1 Q (l/min)"=w518, "Carrier_2 Q (l/min)"=w519, "Trace Gas Concentration (%)"=w517) -> (w527:T5)
                    n199 = Build Array("Clean_Air:Hi-Tec:Dem Volt", "GMU:Back_Pressure:Enable") -> (w524:string[])
                    n200 = Build Array(2.0 ("element"), 1.0 ("element")) -> (w523:dbl[])
                    n201 = call "ASYNC_Adam_client.vi"("Values"=w523, "Channel Names"=w524) -> ()  [unwired: 1 in, 2 out]
                  }
                }
              }
              frame "Check VI only" {
              }
            }
          }
          frame #5 {
            w543 = dbl[] [20.0, 0.0, 0.0, 0.0]  # X Offset
            w545 = dbl[] [100.0, 30.0, 15.0, 0.0]  # Z Offset
            n202 = local read "Mix_own_Calib_Gases"() -> (w541:bool)
            n203 = Unbundle By Name(w540) -> ("Start X"=w542:sgl, "Start Z"=w544:sgl)
            n204 = case shown="True" w541 {
              tunnel: w540 -> [_ w549]
              tunnel: w539 -> [_ w548]
              frame False {
              }
              frame True {
                n205 = call "Set_Source.vi"("Source Status"=Client_Source_Status."Using", "Establish Exp Conditions"=FALSE, "Traverse line"=w549, "Simulate/Run"=w548) -> ()  [unwired: 6 out]
              }
            }
            n206 = for {
              tunnel: w539 -> [w554]
              tunnel: w540 -> [w568]
              tunnel: w545 -> [w567] mode=indexing
              tunnel: w544 -> [w565]
              tunnel: w543 -> [w564] mode=indexing
              tunnel: w542 -> [w563]
              tunnel: [w551] -> w538
              tunnel: w537 -> [w550]
              i -> [w560]
              n207 = Greater?(x=w560, y=1) -> (0:w559:bool)
              n208 = Add(x=w563, y=w564) -> (x+y=w562:dbl)
              n209 = Add(x=w565, y=w567) -> (x+y=w566:dbl)
              n210 = case shown="True" w559 {
                tunnel: ["" "No Backlash"] -> w558
                tunnel: [1.0 ("f") 0.1 ("t")] -> w557
                frame False {
                }
                frame True {
                }
              }
              n211 = Bundle By Name(cluster=w568, "Start X"=w562, "Start Z"=w566, "Specific Arguments"=w558) -> (w556:T5)
              n212 = call "Set_Traverse_Position.vi"("Currently on Point"=1, "Simulate/Run"=w554, "Traverse line"=w556) -> ("Status Cluster"=w555:T23)  [unwired: 3 in]
              n213 = Unbundle By Name(w555) -> ("Status"=w552:T2)
              n214 = global write "Trav_pos_global.vi" "Speed Factor"(w557) -> ()
              n215 = local write "Status"(w552) -> ()
              n216 = call "Prog_Status_Handler.vi"("Status Cluster"=w555, "Simulate/Run"=w554) -> ()  [unwired: 2 out]
              n217 = case shown="Default" w552 {
                tunnel: [w569 Auto_Calib_Case."Skip Next Frame?" ("Currently in Case")] -> w551
                tunnel: w550 -> [w569 _]
                frame "Continue" {
                }
                frame Default {
                }
              }
            }
          }
          frame #6 {
            n218 = global write "Trav_pos_global.vi" "Speed Factor"(1.0 ("Speed Factor")) -> ()
            n219 = case shown="\"Run VI\"" w576 {
              frame "Check VI only", Default {
              }
              frame "Run VI" {
                n220 = while {
                  shift-right: [w588] -> _
                  shift-left: _ -> [w589]
                  tunnel: [w587] -> w582
                  stop <- TRUE stop-if-true
                  n221 = Get Date/Time In Seconds() -> (seconds since 1Jan1904=w588:timestamp)
                  n222 = Subtract(x=w588, y=w589) -> (x-y=w587:dbl)
                }
                n223 = Divide(x=w582, y=3600.0) -> (x/y=w581:dbl)
                n224 = Multiply(x=w581, y=0.2) -> (x*y=w579:dbl)
                n225 = Add(x=w579, y=0.8) -> (x+y=w577:dbl)
                n226 = In Range and Coerce(upper limit=2.0, x=w577, lower limit=1.0) -> (coerced(x)=→"Wait factor":dbl)  [unwired: 1 out]
              }
            }
          }
          frame #7 {
            n227 = local read "Mix_own_Calib_Gases"() -> (w592:bool)
            n228 = case shown="True" w592 {
              tunnel: w594 -> [w603 _]
              tunnel: [w595 0.0] -> w591
              frame False {
                n229 = Tick Count (ms)() -> (millisecond timer value=w602:u32)
                n230 = Subtract(x=w602, y=w603) -> (x-y=w601:u32)
                n231 = local read "Wait factor"() -> (w598:dbl)
                n232 = Divide(x=w601, y=u32 1000) -> (x/y=w597:dbl)
                n233 = Multiply(x=w598, y=20.0) -> (x*y=w596:dbl)
                n234 = Subtract(x=w596, y=w597) -> (x-y=w595:dbl)
              }
              frame True {
              }
            }
            n235 = Greater Than 0?(x=w591) -> (x > 0?=w593:bool)
            n236 = case shown="True" w593 {
              tunnel: w591 -> [_ w606]
              frame False {
              }
              frame True {
                n237 = call "Wait_Seconds_with_display.vi"("Message"="Establishing Exp Conditions", "Seconds to wait"=w606) -> ()  [unwired: 1 in, 1 out]
              }
            }
          }
        }
      }
      frame "Are There Enough Calibration Points" {
        n238 = Array Size(array=w617) -> (size(s)=w618:i32[])
        n239 = Index Array(array=w618, index=0 ("Index")) -> (element=w613:i32)
        "No of Calib Points" <- w613
        n240 = Greater?(x=w613, y=1) -> (0:w614:bool)
        n241 = case shown="True" w614 {
          tunnel: ["Less than two calibration points have been specified\n" ""] -> w610
          tunnel: [Auto_Calib_Case."End" ("Currently in Case") w622] -> w608
          tunnel: w607 -> [_ w622]
          frame False {
          }
          frame True {
          }
        }
        n242 = Concatenate Strings(w612, w610) -> (w611:string)
        "Currently On" <- 1 ("Currently On")
      }
      frame "Set Measurement Conditions" {
        n243 = local read "Currently On"() -> (w628:i32)
        n244 = Decrement(x=w628) -> (x-1=w643:i32)
        n245 = Index Array(array=w644, index (row)=w643) -> (element=w642:dbl[])  [unwired: 1 in]
        n246 = case shown="\"Traverse Position\"" w632 {
          tunnel: w642 -> [w667 w684 w696]
          tunnel: w640 -> [_ _ w693]
          tunnel: w645 -> [w665 w680 w699]
          tunnel: [w666 w679 w691] -> w626
          tunnel: w628 -> [w662 _ w690]
          tunnel: w627 -> [_ _ w689]
          tunnel: [0.0 ("f") 5.0 ("f") w688] -> w624
          frame "Tunnel Speed" {
            n247 = Index Array(array=w667, index=0 ("Index")) -> (element=w655:dbl)
            n248 = while {
              shift-right: [w675] -> w657
              shift-left: _ -> [w674]
              tunnel: w655 -> [w677]
              tunnel: [w675] -> w664
              tunnel: [w674] -> w663
              stop <- FALSE continue-if-true
              n249 = Greater Than 0?(x=w677) -> (x > 0?=w675:bool)
            }
            n250 = Exclusive Or(1:w663, 2:w664) -> (0:w660:bool)
            n251 = Greater?(x=w662, y=1) -> (0:w659:bool)
            n252 = And(x=w660, y=w659) -> (x .and. y?=w658:bool)
            n253 = case shown="False" w657 {
              tunnel: [w669 w671] -> w656
              tunnel: w655 -> [w670 w671]
              frame False {
                n254 = Negate(x=w670) -> (-x=w669:dbl)
              }
              frame True {
              }
            }
            n255 = case shown="False" w658 {
              frame False {
              }
              frame True {
                n256 = call "Wait_Seconds_with_display.vi"("Message"="Please rotate the probe you are calibrating", "Seconds to wait"=10000.0) -> ()  [unwired: 2 out]
              }
            }
            n257 = Bundle By Name(cluster=w665, "Tunnel Speed"=w656) -> (w666:T5)
          }
          frame "Traverse Position" {
            n258 = Index Array(array=w684, index=0 ("Index")) -> (element=w683:dbl)
            n259 = Index Array(array=w684, index=1 ("Index")) -> (element=w682:dbl)
            n260 = Index Array(array=w684, index=2 ("Index")) -> (element=w681:dbl)
            n261 = Bundle By Name(cluster=w680, "Start X"=w683, "Start Y"=w682, "Start Z"=w681) -> (w679:T5)
          }
          frame "Concentration" {
            w698 = nan ("Start X")
            n262 = local read "Mix_own_Calib_Gases"() -> (w697:bool)
            n263 = Bundle By Name(cluster=w699, "Start X"=w698, "Start Y"=w698, "Start Z"=w698) -> (w692:T5)
            n264 = case shown="True" w697 {
              tunnel: w696 -> [w709 w725]
              tunnel: [w708 4.0] -> w695
              tunnel: w692 -> [w707 w722]
              tunnel: [w707 w723] -> w691
              tunnel: [w704 w716] -> w688
              tunnel: w690 -> [w703 _]
              tunnel: w689 -> [_ w720]
              frame False {
                n265 = Index Array(array=w709) -> (element=w708:dbl)  [unwired: 1 in]
                n266 = case shown="3" w703 {
                  tunnel: [0.0 20.0 20.0] -> w705
                  frame 1 {
                  }
                  frame 2, Default {
                  }
                  frame 3 {
                  }
                }
                n267 = local read "Wait factor"() -> (w706:dbl)
                n268 = Multiply(x=w706, y=w705) -> (x*y=w704:dbl)
              }
              frame True {
                n269 = Index Array(array=w725) -> (element #1=w713:dbl, element #2=w714:dbl, element #3=w715:dbl)  [unwired: 3 in]
                n270 = Subtract(x=30.0, y=w720) -> (x-y=w718:dbl)
                n271 = Bundle By Name(cluster=w722, "Carrier_1 Q (l/min)"=w713, "Carrier_2 Q (l/min)"=w714, "Trace Gas Concentration (%)"=w715) -> (w723:T5)
                n272 = Greater Than 0?(x=w718) -> (x > 0?=w719:bool)
                n273 = Select(t=w718, s=w719, f=0.0) -> (s? t:f=w716:dbl)
              }
            }
            n274 = case shown="\"Run VI\"" w693 {
              tunnel: w695 -> [w700 w702]
              tunnel: [w700 w701] -> w694
              frame "Check VI only" {
              }
              frame "Run VI" {
                n275 = call "Fast_FID_Valve_Control.vi"("Requested Position"=w702) -> ("Achieved Posn."=w701:T22)  [unwired: 6 out]
              }
            }
            "Valve position" <- w694
          }
        }
        n276 = stacked-sequence {
          tunnel: w640 -> [w648 w650]
          tunnel: w626 -> [w647 _]
          tunnel: [w646 _] -> w625
          tunnel: w624 -> [_ w651]
          frame #0 {
            n277 = call "Set_Measurement_Conditions.vi"("Simulate/Run"=w648, "Currently on Point"=1, "Traverse line"=w647) -> ("Status Cluster"=w646:T23)  [unwired: 2 out]
          }
          frame #1 {
            n278 = case shown="\"Run VI\"" w650 {
              tunnel: w651 -> [_ w653]
              frame "Check VI only" {
              }
              frame "Run VI" {
                n279 = call "Wait_Seconds_with_display.vi"("Message"="Establishing Calibration Conditions", "Seconds to wait"=w653) -> ()  [unwired: 1 in, 1 out]
              }
            }
          }
        }
        n280 = Unbundle By Name(w625) -> ("Status"=w631:T2)
        "Status" <- w631
        n281 = Equal?(x=w631, y=Multi_Run_Status."Continue" ("Status")) -> (x = y?=w636:bool)
        n282 = Equal?(x=User_Specific_mode."Run VI" ("Mode"), y=w640) -> (x = y?=w637:bool)
        n283 = Increment(x=w629) -> (x+1=w634:T1)
        n284 = And(x=w636, y=w637) -> (x .and. y?=w635:bool)
        n285 = Select(t=w629, s=w635, f=w634) -> (s? t:f=w633:T1)
      }
      frame "Measure Calibration Point" {
        n286 = local read "Mix_own_Calib_Gases"() -> (w726:bool)
        n287 = case shown="\"Concentration\"" w733 {
          tunnel: w732 -> [_ w743]
          tunnel: [w736 w742] -> w728
          tunnel: [w734 w741] -> w727
          tunnel: w726 -> [_ w740]
          frame "Tunnel Speed", Default {
            n288 = local read "New Calib Filenames"() -> (w737:path[])
            n289 = Index Array(array=w737, index=0 ("Index")) -> (element=w738:path)
            n290 = call "Calibration.vi"("Mode"=Calib_mode."Take a New Calibration Point", "Calib file"=w738) -> ("Coefficients"=w734:dbl[][], "Status Out"=w736:T2)  [unwired: 1 in, 15 out]
          }
          frame "Concentration" {
            # "St Dev"
            # "Mean"
            n291 = stacked-sequence {
              seq-local: [_ w749 _] -> [_ _ w816]
              seq-local: [_ w748 _] -> [_ _ w815]
              seq-local: [_ w746 _] -> [_ _ w813]
              tunnel: w743 -> [_ w752 _]
              tunnel: [_ w750 _] -> w742
              tunnel: [_ _ w817] -> w741
              tunnel: w740 -> [_ w747 w814]
              frame #0 {
                n292 = global write "Meas_global.vi" "Remote control"(TRUE ("Remote control")) -> ()
                n293 = global write "Meas_global.vi" "Raw data option"(enum16{"Save raw data", "Raw data not saved"}."Save raw data" ("Raw data option")) -> ()
              }
              frame #1 {
                n294 = local read "New Calib Filenames"() -> (w753:path[])
                n295 = Index Array(array=w753, index=0 ("Index")) -> (element=w751:path)
                n296 = while {
                  tunnel: [w763] -> w750
                  tunnel: w751 -> [w762]
                  tunnel: w752 -> [w760]
                  tunnel: [w759] -> w749
                  tunnel: [w758] -> w748
                  tunnel: w747 -> [w756]
                  tunnel: [w755] -> w746
                  i -> [w757]
                  stop <- w761 continue-if-true
                  n297 = stacked-sequence {
                    seq-local: [_ w767 _ _] -> [_ _ _ w806]
                    seq-local: [_ _ w776 _] -> [_ _ _ w810]
                    seq-local: [_ _ w774 _] -> [_ _ _ w802]
                    tunnel: [_ w767 _ _] -> w763
                    tunnel: w762 -> [_ w771 _ _]
                    tunnel: [_ _ _ w803] -> w761
                    tunnel: w760 -> [_ w768 _ _]
                    tunnel: [_ _ w777 _] -> w759
                    tunnel: [_ _ w776 _] -> w758
                    tunnel: w757 -> [_ _ _ w808]
                    tunnel: w756 -> [_ _ _ w794]
                    tunnel: [_ w765 _ _] -> w755
                    frame #0 {
                      n298 = global write "Meas_global.vi" "Remote control"(TRUE ("Remote control")) -> ()
                    }
                    frame #1 {
                      n299 = call "Get_Data_Base_file_code.vi"("Data Type"="Raw_Calibrations", "Results Filename"=w771, "Short_Name"="Raw_Cal" ("Data Type")) -> ("Raw Data File Name"=w765:path)  [unwired: 1 in, 3 out]
                      n300 = call "Measurement.vi"("setup"=Setup."Run Program", "Post Process"=Post_Process."Take New Data", "File"=Save_Data."Save No Data", "Raw data file"=w765, "Setup filename"=w768) -> ("Status Out"=w767:T2)  [unwired: 2 in, 12 out]
                    }
                    frame #2 {
                      n301 = local read "FF Indexes"() -> (w778:i16[])
                      n302 = global read "Meas_global.vi" "Time Trace"() -> (w775:T24[])
                      n303 = for {
                        tunnel: w778 -> [w791] mode=indexing
                        tunnel: [w790] -> w777 mode=indexing
                        tunnel: [w789] -> w776 mode=indexing
                        tunnel: w775 -> [w787]
                        tunnel: [w780] -> w774 mode=indexing
                        n304 = Index Array(array=w787, index=w791) -> (element=w786:T24)
                        n305 = Unbundle By Name(w786) -> ("Eng Values"=w779:dbl[], "Time (s)"=w785:dbl[])
                        n306 = call-poly <vilib>:"Mean.vi"("X"=w779) -> ("mean"=w783:dbl)  [unwired: 1 out]
                        n307 = Max & Min(x=w783, y=0.3) -> (max(x,y)=w781:dbl)  [unwired: 1 out]
                        n308 = Divide(x=w779, y=w781) -> (x/y=w784:dbl[])
                        n309 = call <vilib>:"Linear Fit.vi"("Y"=w784, "X"=w785) -> ("slope"=w780:dbl)  [unwired: 9 in, 4 out]
                        n310 = call "De-spiked_Stats.vi"("Raw Signal"=w779, "No of st dev to chop at"=6.0) -> ("mean"=w790:dbl, "standard deviation"=w789:dbl)  [unwired: 1 out]
                      }
                    }
                    frame #3 {
                      n311 = Select(t=0.0002, s=w794, f=6e-05) -> (s? t:f=w792:dbl)
                      n312 = Absolute Value(x=w802) -> (abs(x)=w799:dbl[])
                      n313 = Greater?(x=w799, y=w792) -> (0:w800:bool[])
                      n314 = Greater?(x=w810, y=0.15) -> (0:w809:bool[])
                      n315 = Or Array Elements(Boolean array=w800) -> (logical OR=w797:bool)
                      n316 = Or Array Elements(Boolean array=w809) -> (logical OR=w796:bool)
                      n317 = Less?(x=w808, y=4) -> (x < y?=w804:bool)
                      n318 = Equal?(x=w806, y=Multi_Run_Status."Continue" ("Status Out")) -> (x = y?=w801:bool)
                      n319 = Or(x=w797, y=w796) -> (x .or. y?=w798:bool)
                      n320 = Compound Arithmetic op=AND(w801, w798, w804) -> (w803:bool)
                      "Slope" <- w802
                    }
                  }
                }
              }
              frame #2 {
                n321 = case shown="False" w814 {
                  tunnel: [w826 w836] -> w822
                  tunnel: w813 -> [_ w840]
                  tunnel: [nan w828] -> w812
                  frame False {
                    n322 = local read "Valve position"() -> (w827:dbl)
                    n323 = local read "Concentrations"() -> (w825:dbl[])
                    n324 = Index Array(array=w825, index=w827) -> (element=w826:dbl)
                  }
                  frame True {
                    n325 = call "Read_RD_Ch_header.vi"("Raw data file"=w840) -> ("Ch Name Out"=w829:string[], "Ch Values"=w830:string[])  [unwired: 2 out]
                    n326 = Search 1D Array(1D array=w829, element="GMU:Source:Meas Strength") -> (index of element=w838:i32)  [unwired: 1 in]
                    n327 = Search 1D Array(1D array=w829, element="GMU:Source:ppm/%Density") -> (index of element=w832:i32)  [unwired: 1 in]
                    n328 = Index Array(array=w830, index=w838) -> (element=w837:string)
                    n329 = Index Array(array=w830, index=w832) -> (element=w833:string)
                    n330 = Fract/Exp String To Number(string=w837) -> (number=w835:dbl)  [unwired: 3 in, 1 out]
                    n331 = Fract/Exp String To Number(string=w833) -> (number=w828:dbl)  [unwired: 3 in, 1 out]
                    n332 = Multiply(x=10000.0, y=w835) -> (x*y=w836:dbl)
                  }
                }
                n333 = local read "FFID St Dev"() -> (w819:dbl[][])
                n334 = Build Array (concatenate)(w816, w815) -> (w818:dbl[])
                n335 = Build Array (concatenate)(w819, w818) -> (→"FFID St Dev":dbl[][])
                n336 = global read "Meas_global.vi" "Temp"() -> (w823:dbl)
                n337 = local read "New Calib Filenames"() -> (w821:path[])
                n338 = for {
                  tunnel: w816 -> [w847] mode=indexing
                  tunnel: w823 -> [w846]
                  tunnel: w822 -> [w845]
                  tunnel: [w844] -> w817 mode=indexing
                  tunnel: w821 -> [w843] mode=indexing
                  tunnel: w815 -> [w842] mode=indexing
                  tunnel: w812 -> [w841]
                  n339 = stacked-sequence {
                    tunnel: w847 -> [w853 _]
                    tunnel: w846 -> [w850 _]
                    tunnel: w845 -> [w852 _]
                    tunnel: [_ w855] -> w844
                    tunnel: w843 -> [_ w854]
                    tunnel: w842 -> [w849 _]
                    tunnel: w841 -> [w848 _]
                    frame #0 {
                      n340 = Build Array(w852, w853, w849, w848, w850) -> (w851:dbl[])
                      n341 = global write "Calib_global.vi" "Calibration Points"(w851) -> ()
                    }
                    frame #1 {
                      n342 = call "Calibration.vi"("Mode"=Calib_mode."Refit Curve", "Calib file"=w854) -> ("Coefficients"=w856:dbl[][])  [unwired: 1 in, 16 out]
                      n343 = Index Array(array=w856, index (row)=0 ("Index")) -> (element=w855:dbl[])  [unwired: 1 in]
                    }
                  }
                }
              }
            }
          }
        }
        "Coefficients" <- w727
        n344 = local write "Status"(w728) -> ()
      }
      frame "Do Another Calibration Point?" {
        n345 = local read "No of Calib Points"() -> (w872:i32)
        n346 = local read "Status"() -> (w868:T2)
        n347 = local read "Currently On"() -> (w864:i32)
        n348 = case shown="\"Terminate Run\"" w868 {
          tunnel: [w882 w883 TRUE w886] -> w870
          tunnel: [w882 w883 FALSE w886] -> w871
          frame "Continue", Default {
            w882 = TRUE
          }
          frame "Jump to Next Point" {
            w883 = TRUE
          }
          frame "Jump to Next Row" {
          }
          frame "Terminate Run" {
            w886 = FALSE
          }
        }
        n349 = Greater?(x=w872, y=w864) -> (0:w869:bool)
        n350 = Compound Arithmetic op=AND(invert "stop", w870) -> (w867:bool)
        n351 = Compound Arithmetic op=AND(w867, w871, w869) -> (w865:bool)
        n352 = case shown="False" w865 {
          tunnel: w864 -> [_ w881]
          tunnel: [w875 Auto_Calib_Case."Set Measurement Conditions" ("Currently in Case")] -> w863
          tunnel: w862 -> [w876 _]
          tunnel: w861 -> [w874 _]
          frame False {
            n353 = case shown="\"Run VI\"" w876 {
              tunnel: [Auto_Calib_Case."End" ("Currently in Case") Auto_Calib_Case."Skip Next Frame?" ("Currently in Case")] -> w875
              tunnel: w874 -> [_ _]
              frame "Check VI only" {
              }
              frame "Run VI" {
              }
            }
          }
          frame True {
            n354 = Increment(x=w881) -> (x+1=w880:i32)
            n355 = local write "Currently On"(w880) -> ()
          }
        }
        n356 = case shown="True" "stop" {
          frame False {
          }
          frame True {
            n357 = local write "Status"(Multi_Run_Status."Terminate Run" ("Status")) -> ()
          }
        }
      }
      frame "Skip Next Frame?" {
        n358 = local read "Status"() -> (w891:T2)
        n359 = case shown="\"Concentration\"" w888 {
          tunnel: w887 -> [_ _]
          frame "Tunnel Speed", Default {
          }
          frame "Concentration" {
            w894 = T22 1 items=["", "Zero Air", "Calib 1", "Calib 2", "Measure"] ("Requested Position")
            n360 = call "Fast_FID_Valve_Control.vi"("Requested Position"=w894) -> ()  [unwired: 7 out]
          }
        }
        n361 = case shown="\"Terminate Run\", Default" w891 {
          tunnel: [w895 Auto_Calib_Case."End" ("Currently in Case")] -> w890
          tunnel: w889 -> [w895 _]
          frame "Continue" {
          }
          frame "Terminate Run", Default {
          }
        }
      }
      frame "Insert New calibration Filenames into Measurement Setup file" {
        n362 = local read "New Calib Filenames"() -> (w897:path[])
        n363 = global read "Meas_global.vi" "Raw data file"() -> (w907:path)
        n364 = local read "Ch No's"() -> (w898:i16[])
        n365 = Strip Path(path=w907) -> (stripped path=w906:path)  [unwired: 1 out]
        n366 = Equal?(x=Auto_Calib_Type."Concentration" ("Calibration varying"), y=w904) -> (x = y?=w903:bool)
        n367 = call "Current_Calib_Filenames.vi"("Calib Filename"=w897, "Channel Numbers"=w898, "Mode"=App_Global."Write to Global") -> ()  [unwired: 3 out]
        n368 = case shown="False" w903 {
          tunnel: [Auto_Calib_Case."Warn if Current Calibration fit is poor" ("Currently in Case") w914] -> w902
          tunnel: w901 -> [_ w914]
          tunnel: w897 -> [_ w913]
          tunnel: [1 w912] -> w900
          frame False {
          }
          frame True {
            n369 = Array Size(array=w913) -> (size(s)=w912:i32)
          }
        }
        n370 = for {
          N: w900 -> [_]
          tunnel: w897 -> [w916] mode=indexing
          tunnel: w906 -> [w920]
          w918 = FALSE  # Variable Target?
          n371 = Strip Path(path=w916) -> (name=w919:string)  [unwired: 1 out]
          n372 = Build Path(base path=w920, name or relative path=w919) -> (appended path=w915:path)
          n373 = call "Remember_Calib_Filenames.vi"("Filename to Remember"=w915) -> ()  [unwired: 1 out]
          n374 = call "Copy_with_Check.vi"("Mode"=enum16{"Move", "Copy"}."Copy", "Target Path"=w915, "Variable Target?"=w918, "Source Path"=w916) -> ()  [unwired: 1 out]
        }
      }
      frame "Warn if FFID calibration is very non linear" {
        w937 = FALSE  # Dialog Box (T)
        n375 = local read "Root Name"() -> (w936:string[])
        n376 = local read "Coefficients"() -> (w939:dbl[][])
        n377 = for {
          tunnel: w939 -> [w946] mode=indexing
          shift-right: [w948] -> w934
          shift-left: "" -> [w949]
          tunnel: w936 -> [w950] mode=indexing
          tunnel: [w943] -> w929 mode=indexing
          tunnel: "If the calibration fit for %s had been linear instead of a second order polynomial, it would have yielded an average fit error of %.1f%%.\\n" ("Format String") -> [w941]
          n378 = Index Array(array=w946, index=0 ("Index")) -> (element=w944:dbl)
          n379 = Absolute Value(x=w944) -> (abs(x)=w943:dbl)
          n380 = Less?(x=w943, y=2.2) -> (x < y?=w947:bool)
          n381 = case shown="False" w947 {
            tunnel: w950 -> [w952 _]
            tunnel: w943 -> [w953 _]
            tunnel: w949 -> [w956 w957]
            tunnel: [w954 w957] -> w948
            tunnel: w941 -> [w951 _]
            frame False {
              n382 = Format Into String(format string=w951, w952, w953) -> (resulting string=w955:string)  [unwired: 2 in, 1 out]
              n383 = Concatenate Strings(w956, w955) -> (w954:string)
            }
            frame True {
            }
          }
        }
        n384 = Array Max & Min(array=w929) -> (max value=w928:dbl)  [unwired: 3 out]
        n385 = Greater?(x=w928, y=7.0) -> (0:w926:bool)
        n386 = Select(t="Very Poor FFID Linearity", s=w926, f="Poor FFID Linearity") -> (s? t:f=w923:string)
        n387 = Empty String/Path?(string/path=w934) -> (empty?=w933:bool)
        n388 = Not(x=w933) -> (.not. x?=w932:bool)
        n389 = Bundle By Name(cluster=errorcluster {"status"=FALSE, "code"=0, "source"=""} ("error in (no error)"), "source"=w934, "status"=w932) -> (w931:errorcluster)
        n390 = call "EnFlo_Error_Handler.vi"("error in (no error)"=w931, "Error Type"=w923, "Dialog Box (T)"=w937) -> ()  [unwired: 3 out]
      }
      frame "Warn if FFID variance is high" {
        w979 = FALSE  # Dialog Box (T)
        n391 = local read "New Calib Filenames"() -> (w961:path[])
        n392 = local read "FFID St Dev"() -> (w981:dbl[][])
        n393 = Index Array(array=w966, index (col)=0 ("disabled index (col)")) -> (element=w964:dbl[])  [unwired: 1 in]
        n394 = Array Size(array=w961) -> (size(s)=w960:i32)
        n395 = for {
          tunnel: w981 -> [w998]
          shift-right: [w1000] -> w977
          shift-left: "" -> [w1001]
          tunnel: w961 -> [w989] mode=indexing
          tunnel: "For %s the measurement at %dppm had a standard deviation of %.2f volts for an average value of  %.1f volts.\\n" ("Format String") -> [w999]
          tunnel: w964 -> [w992]
          tunnel: [w991] -> w962 mode=indexing
          tunnel: w960 -> [w987]
          tunnel: [w983] -> w958 mode=indexing
          i -> [w986]
          n396 = Add(x=w987, y=w986) -> (x+y=w985:i32)
          n397 = Strip Path(path=w989) -> (name=w988:string)  [unwired: 1 out]
          n398 = Index Array(array=w998, index (col)=w986) -> (element=w990:dbl[])  [unwired: 1 in]
          n399 = Index Array(array=w998, index (col)=w985) -> (element=w984:dbl[])  [unwired: 1 in]
          n400 = Array Max & Min(array=w984) -> (min value=w983:dbl)  [unwired: 3 out]
          n401 = call-poly <vilib>:"Mean.vi"("X"=w990) -> ("mean"=w997:dbl)  [unwired: 1 out]
          n402 = Divide(x=w984, y=w997) -> (x/y=w996:dbl[])
          n403 = Array Max & Min(array=w996) -> (max value=w991:dbl, max index (indices)=w993:i32)  [unwired: 2 out]
          n404 = Greater?(x=w991, y=0.06) -> (0:w994:bool)
          n405 = case shown="True" w994 {
            tunnel: w988 -> [_ w1012]
            tunnel: w1001 -> [w1002 w1018]
            tunnel: [w1002 w1016] -> w1000
            tunnel: w999 -> [_ w1015]
            tunnel: w993 -> [_ w1013]
            tunnel: w992 -> [_ w1014]
            tunnel: w991 -> [_ _]
            tunnel: w984 -> [_ w1011]
            tunnel: w990 -> [_ w1009]
            frame False {
            }
            frame True {
              n406 = local read "Concentrations"() -> (w1007:dbl[])
              n407 = Index Array(array=w1014, index=w1013) -> (element=w1008:dbl)
              n408 = Index Array(array=w1011, index=w1013) -> (element=w1005:dbl)
              n409 = Index Array(array=w1009, index=w1013) -> (element=w1010:dbl)
              n410 = Index Array(array=w1007, index=w1008) -> (element=w1006:dbl)
              n411 = Multiply(x=w1005, y=2.5) -> (x*y=w1004:dbl)
              n412 = Format Into String(format string=w1015, w1012, w1006, w1004, w1010) -> (resulting string=w1017:string)  [unwired: 2 in, 1 out]
              n413 = Concatenate Strings(w1018, w1017) -> (w1016:string)
            }
          }
        }
        "Minimum St Dev" <- w958
        n414 = Array Max & Min(array=w962) -> (max value=w972:dbl)  [unwired: 3 out]
        n415 = Greater?(x=w972, y=0.09) -> (0:w970:bool)
        n416 = Select(t="Very unstable FFID calibration point", s=w970, f="Unstable FFID calibration point") -> (s? t:f=w967:string)
        n417 = Empty String/Path?(string/path=w977) -> (empty?=w976:bool)
        n418 = Not(x=w976) -> (.not. x?=w975:bool)
        n419 = Bundle By Name(cluster=errorcluster {"status"=FALSE, "code"=0, "source"=""} ("error in (no error)"), "source"=w977, "status"=w975) -> (w974:errorcluster)
        n420 = call "EnFlo_Error_Handler.vi"("error in (no error)"=w974, "Error Type"=w967, "Dialog Box (T)"=w979) -> ()  [unwired: 3 out]
      }
      frame "Insert Bkgnd Variance into calib file" {
        n421 = local read "New Calib Filenames"() -> (w1021:path[])
        n422 = local read "Minimum St Dev"() -> (w1022:dbl[])
        n423 = local read "Coefficients"() -> (w1019:dbl[][])
        n424 = for {
          tunnel: w1022 -> [w1027] mode=indexing
          tunnel: w1021 -> [w1033] mode=indexing
          tunnel: w1019 -> [w1030] mode=indexing
          n425 = call "Read_File_Simple.vi"("Filename"=w1033) -> ("string"=w1037:string)  [unwired: 2 in, 7 out]
          n426 = Index Array(array=w1030, index=2) -> (element=w1028:dbl)
          n427 = Multiply(x=w1027, y=w1028) -> (x*y=w1026:dbl)
          n428 = Square(x=w1026) -> (x^2=w1025:dbl)
          n429 = Number To Fractional String(number=w1025, precision (6)=i16 8) -> (F-format string=w1035:string)  [unwired: 2 out]
          n430 = call "Replace_data_in_setup_string.vi"("New data string"=w1035, "Input string"=w1037, "Variable name"="Fast FID Bkgnd Variance") -> ("Appended string"=w1032:string)
          n431 = call "Write_File_Simple.vi"("append to file? (new file:F)"=FALSE, "character string"=w1032, "file path"=w1033) -> ()  [unwired: 2 out]
        }
      }
      frame "Warn if FFID voltages are too low" {
        w1051 = FALSE  # Dialog Box (T)
        n432 = local read "Coefficients"() -> (w1043:dbl[][])
        n433 = local read "Concentrations"() -> (w1038:dbl[])
        n434 = local read "New Calib Filenames"() -> (w1042:path[])
        n435 = Array Max & Min(array=w1038) -> (max value=w1039:dbl)  [unwired: 3 out]
        n436 = for {
          shift-right: [w1063] -> w1049
          shift-left: "" -> [w1064]
          tunnel: "For %s the maximum measured calibration voltage was %.1f volts.\nCheck that the FID is running and correctly connected to the acquisition system." ("Format String") -> [w1062]
          tunnel: w1043 -> [w1060] mode=indexing
          tunnel: w1042 -> [w1056] mode=indexing
          tunnel: w1039 -> [w1055]
          n437 = Split 1D Array(array=w1060, index=1) -> (second subarray=w1059:dbl[])  [unwired: 1 out]
          n438 = call "Polybackwards.vi"("Coefficients"=w1059, "Y input"=w1055) -> ("X output"=w1054:dbl)  [unwired: 1 out]
          n439 = Less?(x=w1054, y=0.2) -> (x < y?=w1057:bool)
          n440 = case shown="True" w1057 {
            tunnel: w1064 -> [w1065 w1072]
            tunnel: [w1065 w1070] -> w1063
            tunnel: w1062 -> [_ w1069]
            tunnel: w1056 -> [_ w1068]
            tunnel: w1054 -> [_ w1066]
            frame False {
            }
            frame True {
              n441 = Strip Path(path=w1068) -> (name=w1067:string)  [unwired: 1 out]
              n442 = Format Into String(format string=w1069, w1067, w1066) -> (resulting string=w1071:string)  [unwired: 2 in, 1 out]
              n443 = Concatenate Strings(w1072, w1071) -> (w1070:string)
            }
          }
        }
        n444 = Empty String/Path?(string/path=w1049) -> (empty?=w1048:bool)
        n445 = Not(x=w1048) -> (.not. x?=w1047:bool)
        n446 = Bundle By Name(cluster=errorcluster {"status"=FALSE, "code"=0, "source"=""} ("error in (no error)"), "source"=w1049, "status"=w1047) -> (w1046:errorcluster)
        n447 = call "EnFlo_Error_Handler.vi"("error in (no error)"=w1046, "Error Type"="Low FFID calibration voltages", "Dialog Box (T)"=w1051) -> ()  [unwired: 3 out]
      }
      frame "Warn if Current Calibration fit is poor" {
        w1091 = FALSE  # Dialog Box (T)
        n448 = local read "Root Name"() -> (w1090:string[])
        n449 = local read "Coefficients"() -> (w1093:dbl[][])
        n450 = local read "Mix_own_Calib_Gases"() -> (w1075:bool)
        n451 = Select(t=1.5, s=w1075, f=1.0 ("y")) -> (s? t:f=w1073:dbl)
        n452 = for {
          tunnel: w1093 -> [w1100] mode=indexing
          shift-right: [w1102] -> w1088
          shift-left: "" -> [w1103]
          tunnel: w1090 -> [w1104] mode=indexing
          tunnel: [w1097] -> w1083 mode=indexing
          tunnel: w1073 -> [w1096]
          n453 = Index Array(array=w1100, index=0 ("Index")) -> (element=w1098:dbl)
          n454 = Absolute Value(x=w1098) -> (abs(x)=w1097:dbl)
          n455 = Less?(x=w1097, y=w1096) -> (x < y?=w1101:bool)
          n456 = case shown="True" w1101 {
            tunnel: w1104 -> [w1106 _]
            tunnel: w1097 -> [w1107 _]
            tunnel: w1103 -> [w1110 w1111]
            tunnel: [w1108 w1111] -> w1102
            frame False {
              n457 = Format Into String(format string="The calibration for %s has an average fit error of %.1f%%\\n" ("Format String"), w1106, w1107) -> (resulting string=w1109:string)  [unwired: 2 in, 1 out]
              n458 = Concatenate Strings(w1110, w1109) -> (w1108:string)
            }
            frame True {
            }
          }
        }
        n459 = Array Max & Min(array=w1083) -> (max value=w1082:dbl)  [unwired: 3 out]
        n460 = Greater?(x=w1082, y=7.0) -> (0:w1080:bool)
        n461 = Select(t="Very Poor Calibration", s=w1080, f="Poor Calibration") -> (s? t:f=w1077:string)
        n462 = Empty String/Path?(string/path=w1088) -> (empty?=w1087:bool)
        n463 = Not(x=w1087) -> (.not. x?=w1086:bool)
        n464 = Bundle By Name(cluster=errorcluster {"status"=FALSE, "code"=0, "source"=""} ("error in (no error)"), "source"=w1088, "status"=w1086) -> (w1085:errorcluster)
        n465 = call "EnFlo_Error_Handler.vi"("error in (no error)"=w1085, "Error Type"=w1077, "Dialog Box (T)"=w1091) -> ()  [unwired: 3 out]
      }
      frame "Warn if Calibration Coefficients have significantly altered" {
        w1137 = FALSE  # Dialog Box (T)
        w1124 = 8.0 ("y")
        n466 = local read "New Calib Filenames"() -> (w1129:path[])
        n467 = local read "Root Name"() -> (w1128:string[])
        n468 = global read "Calib_global.vi" "Instrument type"() -> (w1127:T15)
        n469 = Unbundle By Name(w1116) -> ("Extra Commands"=w1115:string)
        n470 = global read "Extra_Commands_Global.vi" "If Command"() -> (w1117:string)
        n471 = call "Extra_Commands.vi"("String to Search"=w1115, "Command"=w1117) -> ("String Value"=w1114:string)  [unwired: 1 in, 4 out]
        n472 = call "Calibration_Analysis.vi"("Root Name"=w1128, "New Calib Filenames"=w1129, "Instrument type"=w1127, "Clear Calib History"="Clear Calib History") -> ("Error String"=w1126:string, "Max % Error"=w1112:dbl)
        n473 = call "Get_array_values_fr_String.vi"("String Value"=w1114) -> ("Numeric Array"=w1113:dbl[], "String array"=w1119:string[])
        n474 = Greater?(x=w1112, y=w1124) -> (0:w1125:bool)
        n475 = Index Array(array=w1119, index=0 ("Index")) -> (element=w1120:string)
        n476 = case shown="\"Drift Greater Than\"" w1120 {
          tunnel: w1113 -> [w1143 _]
          tunnel: w1112 -> [w1142 _]
          frame "Drift Greater Than" {
            n477 = Index Array(array=w1143, index=1 ("Index")) -> (element=w1141:dbl)
            n478 = Greater?(x=w1142, y=w1141) -> (0:w1140:bool)
            n479 = case shown="True" w1140 {
              frame False {
              }
              frame True {
                n480 = local write "Status"(Multi_Run_Status."Jump To Fall Back" ("Status")) -> ()
              }
            }
          }
          frame "No Match", Default {
          }
        }
        n481 = Format Into String(format string="Calibration Drift Greater than %d%%", w1124) -> (resulting string=w1122:string)  [unwired: 2 in, 1 out]
        n482 = Select(t=w1122, s=w1125, f="Calibration Drift") -> (s? t:f=w1130:string)
        n483 = Empty String/Path?(string/path=w1126) -> (empty?=w1135:bool)
        n484 = Not(x=w1135) -> (.not. x?=w1134:bool)
        n485 = Bundle By Name(cluster=errorcluster {"status"=FALSE, "code"=0, "source"=""} ("error in (no error)"), "source"=w1126, "status"=w1134) -> (w1133:errorcluster)
        n486 = call "EnFlo_Error_Handler.vi"("error in (no error)"=w1133, "Error Type"=w1130, "Dialog Box (T)"=w1137) -> ()  [unwired: 3 out]
      }
      frame "End" {
        n487 = case shown="\"Concentration\"" w1149 {
          tunnel: w1147 -> [_ w1155]
          tunnel: w1148 -> [_ w1154]
          tunnel: w1146 -> [_ w1153]
          frame "Tunnel Speed", Default {
          }
          frame "Concentration" {
            n488 = stacked-sequence {
              tunnel: w1155 -> [w1171 _]
              tunnel: w1154 -> [w1163 w1178]
              tunnel: w1153 -> [w1157 _]
              frame #0 {
                n489 = Unbundle By Name(w1171) -> ("Averaging time (min)"=w1173:dbl)
                n490 = global read "Trav_pos_global.vi" "Simulation Time"() -> (w1166:timestamp)
                n491 = Unbundle By Name(w1171) -> ("Start X"=w1161:sgl, "Start Z"=w1162:sgl)
                n492 = Array Size(array=w1157) -> (size(s)=w1158:i32[])
                n493 = Index Array(array=w1158) -> (element=w1156:i32)  [unwired: 1 in]
                n494 = Multiply(x=60.0, y=w1173) -> (x*y=w1170:dbl)
                n495 = Add(x=w1161, y=6.0) -> (x+y=w1160:dbl)
                n496 = Add(x=w1162, y=150.0) -> (x+y=w1174:dbl)
                n497 = Add(x=w1170, y=60.0) -> (x+y=w1168:dbl)
                n498 = Bundle By Name(cluster=w1171, "Start X"=w1160, "Start Z"=w1174) -> (w1175:T5)
                n499 = Multiply(x=w1168, y=w1156) -> (x*y=w1167:dbl)
                n500 = Add(x=w1166, y=w1167) -> (x+y=w1164:timestamp)
                n501 = call "Set_Traverse_Position.vi"("Currently on Point"=1, "Simulate/Run"=w1163, "Traverse line"=w1175) -> ()  [unwired: 3 in, 1 out]
                n502 = call "Run_FFID_Bkgnd.vi"("Simulated Time"=w1164, "Run Now?"=TRUE, "Simulate/Run"=w1163) -> ()  [unwired: 3 out]
              }
              frame #1 {
                n503 = case shown="\"Run VI\"" w1178 {
                  frame "Check VI only", Default {
                  }
                  frame "Run VI" {
                    w1180 = T22 4 items=["", "Zero Air", "Calib 1", "Calib 2", "Measure"] ("Requested Position")
                    n504 = local read "Mix_own_Calib_Gases"() -> (w1179:bool)
                    n505 = case shown="True" w1179 {
                      frame False {
                      }
                      frame True {
                        w1182 = 0.0 ("element")
                        n506 = Build Array("Clean_Air:Hi-Tec:Dem Volt", "GMU:Back_Pressure:Enable") -> (w1184:string[])
                        n507 = Build Array(w1182, w1182) -> (w1183:dbl[])
                        n508 = call "ASYNC_Adam_client.vi"("Values"=w1183, "Channel Names"=w1184) -> ()  [unwired: 1 in, 2 out]
                      }
                    }
                    n509 = call "Fast_FID_Valve_Control.vi"("Requested Position"=w1180) -> ()  [unwired: 7 out]
                  }
                }
              }
            }
          }
        }
      }
    }
    "Currently in Case" <- w18
  }
  "Error Messages" <- w12
